vi "Pump Settings Dialog.vi"(8 "error in (no error)":errorcluster, 10 "Message Queues":T17, 11 "Pump Module State Cluster In":T1={"Pump Module Config"={"GUID"="", "Drop Coords"={"Horizontal"=0, "Vertical"=0}, "Process Name"="", "Queue Name"="", "Settings"={"Cycle Period"=500.0, "Manual Entry"=0.0, "Output Device"=enum."Default", "Ismatech"={"VISA resource name"="", "Simulated?"=TRUE, "Pump Number"=1.0, "Reverse?"=FALSE}, "Ismatech 3 Channel Settings"={"VISA resource name"="", "Pump Number"=1, "Channel Number"=0, "Simulated?"=TRUE, "Reverse?"=FALSE}, "Masterflex"={"VISA resource name"="", "Simulated?"=TRUE, "Pump Number"=1.0, "Reverse?"=FALSE}, "VICI Settings"={"VISA resource name"="", "Simulated?"=TRUE, "Pump Letter"="", "Reverse?"=FALSE}, "Tacmina Settings"={"Analog DAQ Task"="", "Digital DAQ Task"=""}, "KNF SIMDOS Settings"={"VISA resource name"="", "Simulated?"=TRUE}, "ASIA Pump C"={"ASIA Pump #"=0, "channel"=0, "Simulated"=FALSE}, "FLOM Settings"={"VISA resource name"="", "Simulated?"=TRUE, "Pump Number"=0.0}, "SSI PR/LD Settings"={"VISA resource name"="", "Simulated?"=FALSE}, "SSI P40 Settings"={"VISA resource name"="", "Simulated?"=FALSE}, "Masterflex 75211 Settings"={"Analog DAQ Task"="", "Digital DAQ Task"=""}, "Pump Calibration File"=path "", "Calibration Slope"=0.0, "Calibration Y Intercept"=0.0, "Pump Cal Enum"=0}, "Load Count"=0}, "State"=enum."Idle", "Start Time"=timestamp(0 s since 1904-01-01), "Current Time"=timestamp(0 s since 1904-01-01), "First Iteration"=FALSE, "Data"={"Pump Speed"=0.0}, "Process Name"="", "Pump On?"=FALSE} {"Pump Module Config"."Settings"."Ismatech 3 Channel Settings"."Channel Number" min=0 max=3; "Pump Module Config"."Settings"."Ismatech 3 Channel Settings"."Pump Number" min=1; "Pump Module Config"."Settings"."ASIA Pump C"."channel" min=0 max=1 step=1; "Pump Module Config"."Settings"."Masterflex"."Pump Number" min=1.0 max=20.0 step=1.0; "Pump Module Config"."Settings"."Ismatech"."Pump Number" min=1.0 max=20.0 step=1.0}) -> (0 "error out":errorcluster, 1 "Cancelled?":bool=TRUE, 2 "UI Refresh Needed?":bool, 3 "Pump Module Config Out":T2={"GUID"="", "Drop Coords"={"Horizontal"=0, "Vertical"=0}, "Process Name"="", "Queue Name"="", "Settings"={"Cycle Period"=0.0, "Manual Entry"=0.0, "Output Device"=enum."Default", "Ismatech"={"VISA resource name"="", "Simulated?"=FALSE, "Pump Number"=0.0, "Reverse?"=FALSE}, "Ismatech 3 Channel Settings"={"VISA resource name"="", "Pump Number"=1, "Channel Number"=0, "Simulated?"=TRUE, "Reverse?"=FALSE}, "Masterflex"={"VISA resource name"="", "Simulated?"=FALSE, "Pump Number"=0.0, "Reverse?"=FALSE}, "VICI Settings"={"VISA resource name"="", "Simulated?"=FALSE, "Pump Letter"="", "Reverse?"=FALSE}, "Tacmina Settings"={"Analog DAQ Task"="", "Digital DAQ Task"=""}, "KNF SIMDOS Settings"={"VISA resource name"="", "Simulated?"=TRUE}, "ASIA Pump C"={"ASIA Pump #"=0, "channel"=0, "Simulated"=FALSE}, "FLOM Settings"={"VISA resource name"="", "Simulated?"=TRUE, "Pump Number"=0.0}, "SSI PR/LD Settings"={"VISA resource name"="", "Simulated?"=FALSE}, "SSI P40 Settings"={"VISA resource name"="", "Simulated?"=FALSE}, "Masterflex 75211 Settings"={"Analog DAQ Task"="", "Digital DAQ Task"=""}, "Pump Calibration File"=path "", "Calibration Slope"=0.0, "Calibration Y Intercept"=0.0, "Pump Cal Enum"=0}, "Load Count"=0} {"Settings"."Ismatech 3 Channel Settings"."Channel Number" min=0 max=3; "Settings"."Ismatech 3 Channel Settings"."Pump Number" min=1; "Settings"."ASIA Pump C"."channel" min=0 max=1 step=1; "Settings"."Masterflex"."Pump Number" min=1.0 max=20.0 step=1.0; "Settings"."Ismatech"."Pump Number" min=1.0 max=20.0 step=1.0})   [LabVIEW 2018, in "Pump Module.lvlib"]
doc: "Dialog for selecting user specified settings."
uses:
  Pump Module.lvlib
  Pump Dialog Config and Start Stop Buttons.ctl
  Ismatec ISM 831C/Controls/Ismatech ISM831C Settings Cluster.ctl
  Masterflex 7550-30/Controls/Settings Cluster.ctl
  VICI M50 Party Mode/Settings Cluster.ctl
  Measure Instrument/PID 2 Output Enum.ctl
  Tacmina QI/Tacmina QI DAQ Setting.ctl
  KNF Pump/Settings Cluster plus SIMDOS.ctl
  ASIA Pump/Pump Settings.ctl
  FLOM Pump/Settings Cluster.ctl
  SSI PR Class/SSI PR or LD Settings Cluster.ctl
  Masterflex 75211/Masterflex 75211 DAQ Setting.ctl
  SSI PR Class/SSI P40 Settings Cluster.ctl
  Ismatec 78001/Ismatec 4083.ctl
  All Message Queues.ctl
  support/Message Queue/Message Cluster.ctl
  Pump Module Config Cluster.ctl
  <vilib>/Utility/miscctls.llb/LVPoint32TypeDef.ctl
  Pump Module Settings Cluster.ctl
  Pump Module State Cluster.ctl
  Measure Instrument/State Enum.ctl
  support/Message Queue/Enqueue Message (Single).vi
  <vilib>/Utility/xml.llb/Write to XML File(string).vi
  <vilib>/Utility/file.llb/Read Delimited Spreadsheet (string).vi
  Settings/Settings.lvlib
  support/Support Library.lvlib
  Masterflex 7550-30/Masterflex 7550-30.lvlib
  Ismatec ISM 831C/Ismatec ISM 831C.lvlib
  Tacmina QI/Tacmina QI.lvlib
  KNF Pump/KNF SIMDOS.lvlib
  VICI M50 Party Mode/VICI M6 M50 Party Mode.lvlib
  support/Message Queue/Message Queue.lvlib
  FLOM Pump/FLOM Pump.lvlib
  SSI PR Class/SSI PR or LD Pump.lvlib
  Masterflex 75211/Masterflex 75211.lvlib
  SSI PR Class/SSI P40 Pump.lvlib
  Ismatec 78001/Ismatec 4308.lvlib
  ASIA Pump.lvlib
  Measure Instrument/Feed Module Engine.lvlib
panel:
  in  "OK Button 2":bool
  in  "Module Name":string
  out "FLOM VISA Chosen":bool
  out "FLOM Number Chosen":bool
  in  "Pump Settings":T18={"Pump Configuration"={"Cycle Period"=500.0, "Ismatech"={"VISA resource name"="", "Simulated?"=FALSE, "Pump Number"=1.0, "Reverse?"=FALSE}, "Masterflex"={"VISA resource name"="", "Simulated?"=FALSE, "Pump Number"=1.0, "Reverse?"=FALSE}, "Pump %"=0.0, "VICI Settings"={"VISA resource name"="", "Simulated?"=FALSE, "Pump Letter"="", "Reverse?"=FALSE}, "Output Device"=enum."Default", "Tacmina Settings"={"Analog DAQ Task"="", "Digital DAQ Task"=""}, "KNF SIMDOS Settings"={"VISA resource name"="", "Simulated?"=FALSE}, "ASIA Pump C"={"ASIA Pump #"=-1, "channel"=-1, "Simulated"=FALSE}, "FLOM Settings"={"VISA resource name"="", "Simulated?"=FALSE, "Pump Number"=1.0}, "Pump Calibration"=0, "SSI PR/LD Settings"={"VISA resource name"="", "Simulated?"=FALSE}, "Masterflex 75211 Settings"={"Analog DAQ Task"="", "Digital DAQ Task"=""}, "SSI P40 Settings"={"VISA resource name"="", "Simulated?"=FALSE}, "Ismatech 3 Channel Settings"={"VISA resource name"="", "Pump Number"=0, "Channel Number"=0, "Simulated?"=FALSE, "Reverse?"=FALSE}}, "Stop"=FALSE, "Start"=FALSE} {"Pump Configuration"."Ismatech 3 Channel Settings"."Channel Number" min=0 max=3; "Pump Configuration"."Ismatech 3 Channel Settings"."Pump Number" min=1; "Pump Configuration"."ASIA Pump C"."channel" min=-1 max=1 step=1; "Pump Configuration"."Ismatech"."Pump Number" min=1.0 max=20.0 step=1.0; "Pump Configuration"."Masterflex"."Pump Number" min=1.0 max=20.0 step=1.0}
  in  "Cancel Button":bool
  in  "OK Button":bool
  # "Non visible portion of dialog (needed for connector pane)."
  # "Output Instruments"
  # "Output Instruments"
  # "Output Instruments"
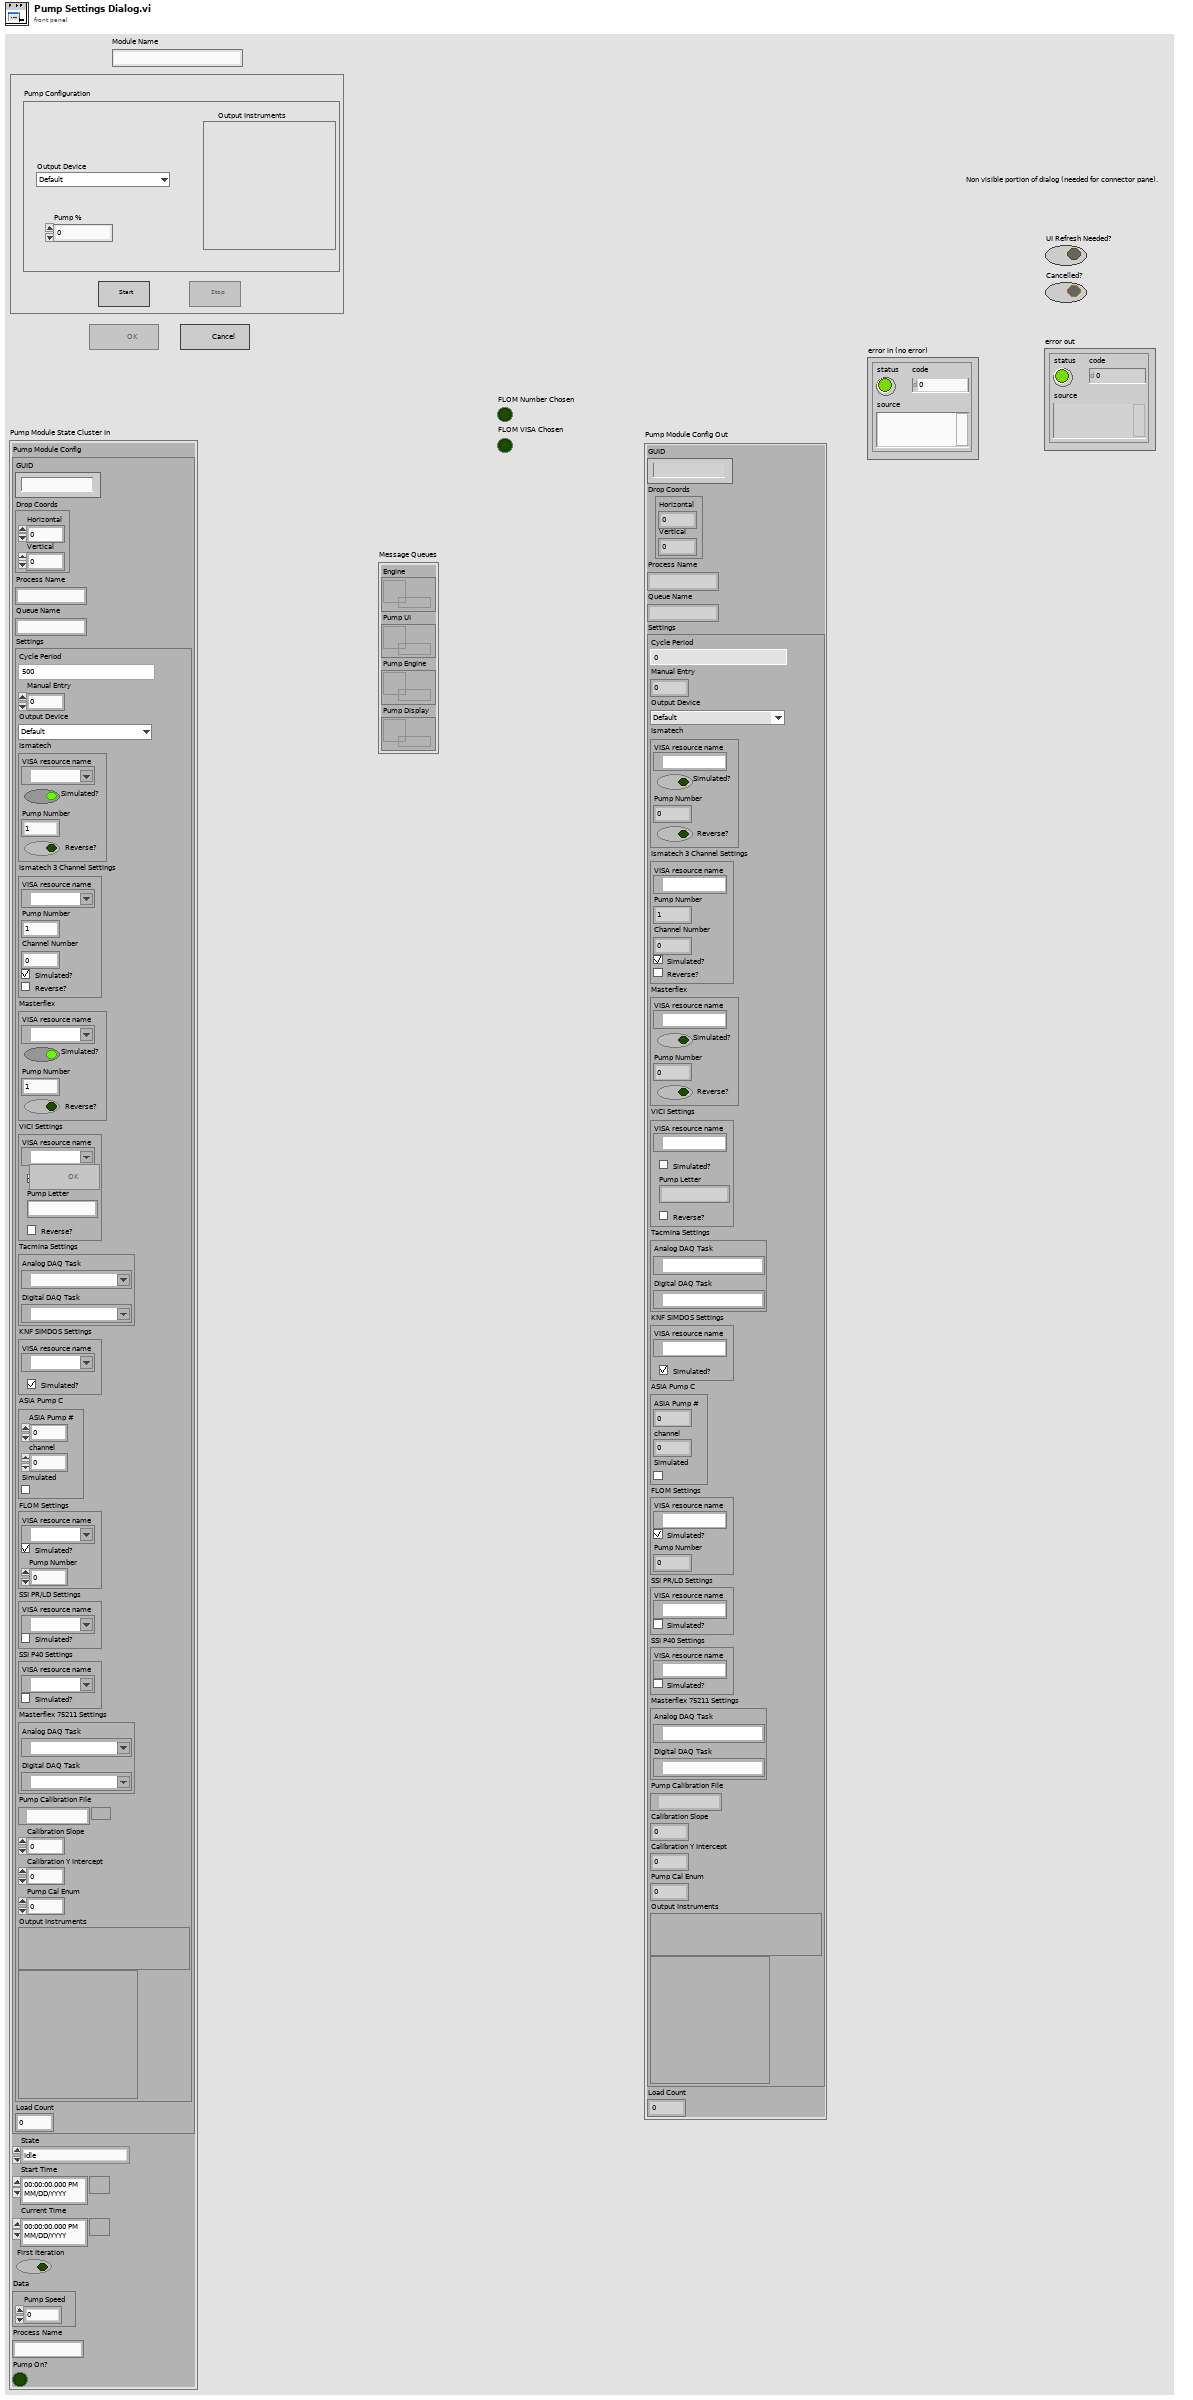
[diagram p1: front panel]
types:
  T1 = typedef "Pump Module.lvlib/Pump Module State Cluster.ctl" = cluster{"Pump Module Config":T2, "State":T16, "Start Time":timestamp, "Current Time":timestamp, "First Iteration":bool, "Data":cluster{"Pump Speed":dbl}, "Process Name":string, "Pump On?":bool}
  T2 = typedef "Pump Module.lvlib/Pump Module Config Cluster.ctl" = cluster{"GUID":string, "Drop Coords":T3, "Process Name":string, "Queue Name":string, "Settings":T4, "Load Count":i32}
  T3 = typedef "LVPoint32TypeDef.ctl" = cluster{"Horizontal":i32, "Vertical":i32}
  T4 = typedef "Pump Module.lvlib/Pump Module Settings Cluster.ctl" = cluster{"Cycle Period":dbl, "Manual Entry":dbl, "Output Device":T5, "Ismatech":T6, "Ismatech 3 Channel Settings":T7, "Masterflex":T8, "VICI Settings":T9, "Tacmina Settings":T10, "KNF SIMDOS Settings":T11, "ASIA Pump C":T12, "FLOM Settings":T13, "SSI PR/LD Settings":T14, "SSI P40 Settings":T14, "Masterflex 75211 Settings":T15, "Pump Calibration File":path, "Calibration Slope":dbl, "Calibration Y Intercept":dbl, "Pump Cal Enum":u16}
  T5 = typedef "PID 2 Output Enum.ctl" = enum16{"Default", "Ismatec ISM 4308", "Ismatec ISM 831C", "Masterflex 7550-30", "VICI", "Tacmina QI", "KNF SIMDOS", "ASIA Type C", "FLOM UI-22-11", "SSI PR/LD", "SSI P40", "Masterflex 75211-70"}
  T6 = typedef "Ismatec ISM 831C.lvlib/Ismatech ISM831C Settings Cluster.ctl" = cluster{"VISA resource name":refnum<visa-resource-name>, "Simulated?":bool, "Pump Number":dbl, "Reverse?":bool}
  T7 = typedef "Ismatec 4308.lvlib/Ismatec 4083.ctl" = cluster{"VISA resource name":refnum<visa-resource-name>, "Pump Number":i16, "Channel Number":i16, "Simulated?":bool, "Reverse?":bool}
  T8 = typedef "Masterflex 7550-30.lvlib/Settings Cluster.ctl" = cluster{"VISA resource name":refnum<visa-resource-name>, "Simulated?":bool, "Pump Number":dbl, "Reverse?":bool}
  T9 = typedef "VICI M6 M50 Party Mode.lvlib/Settings Cluster.ctl" = cluster{"VISA resource name":refnum<visa-resource-name>, "Simulated?":bool, "Pump Letter":string, "Reverse?":bool}
  T10 = typedef "Tacmina QI.lvlib/Tacmina QI DAQ Setting.ctl" = cluster{"Analog DAQ Task":refnum<k21>, "Digital DAQ Task":refnum<k21>}
  T11 = typedef "KNF SIMDOS.lvlib/Settings Cluster plus SIMDOS.ctl" = cluster{"VISA resource name":refnum<visa-resource-name>, "Simulated?":bool}
  T12 = typedef "ASIA Pump.lvlib/Pump Settings.ctl" = cluster{"ASIA Pump #":i32, "channel":i32, "Simulated":bool}
  T13 = typedef "FLOM Pump.lvlib/Settings Cluster.ctl" = cluster{"VISA resource name":refnum<visa-resource-name>, "Simulated?":bool, "Pump Number":dbl}
  T14 = typedef "SSI PR or LD Pump.lvlib/SSI PR or LD Settings Cluster.ctl" = cluster{"VISA resource name":refnum<visa-resource-name>, "Simulated?":bool}
  T15 = typedef "Masterflex 75211.lvlib/Masterflex 75211 DAQ Setting.ctl" = cluster{"Analog DAQ Task":refnum<k21>, "Digital DAQ Task":refnum<k21>}
  T16 = typedef "Feed Module.lvlib/Feed Module Engine.lvlib/State Enum.ctl" = enum16{"Measuring", "Idle", "Paused"}
  T17 = typedef "Pump Module.lvlib/All Message Queues.ctl" = cluster{"Engine":refnum<queue>, "Pump UI":refnum<queue>, "Pump Engine":refnum<queue>, "Pump Display":refnum<queue>}
  T18 = typedef "Pump Module.lvlib/Pump Dialog Config and Start Stop Buttons.ctl" = cluster{"Pump Configuration":cluster{"Cycle Period":dbl, "Ismatech":T6, "Masterflex":T8, "Pump %":dbl, "VICI Settings":T9, "Output Device":T5, "Tacmina Settings":T10, "KNF SIMDOS Settings":T11, "ASIA Pump C":T12, "FLOM Settings":T13, "Pump Calibration":u16, "SSI PR/LD Settings":T14, "Masterflex 75211 Settings":T15, "SSI P40 Settings":T19, "Ismatech 3 Channel Settings":T7}, "Stop":bool, "Start":bool}
  T19 = typedef "SSI P40 Pump.lvlib/SSI P40 Settings Cluster.ctl" = cluster{"VISA resource name":refnum<visa-resource-name>, "Simulated?":bool}
  T20 = cluster{"Cycle Period":dbl, "Ismatech":T6, "Masterflex":T8, "Pump %":dbl, "VICI Settings":T9, "Output Device":T5, "Tacmina Settings":T10, "KNF SIMDOS Settings":T11, "ASIA Pump C":T12, "FLOM Settings":T13, "Pump Calibration":u16, "SSI PR/LD Settings":T14, "Masterflex 75211 Settings":T15, "SSI P40 Settings":T19, "Ismatech 3 Channel Settings":T7}
  T21 = cluster{"Pump Configuration":cluster{"Cycle Period":dbl, "Ismatech":T6, "Masterflex":T8, "Pump %":dbl, "VICI Settings":T9, "Output Device":T5, "Tacmina Settings":T10, "KNF SIMDOS Settings":T11, "ASIA Pump C":T12, "FLOM Settings":T13, "Pump Calibration":u16, "SSI PR/LD Settings":T14, "Masterflex 75211 Settings":T15, "SSI P40 Settings":T19, "Ismatech 3 Channel Settings":T7}, "Stop":bool, "Start":bool}
  T22 = enum8{"Enabled", "Disabled", "Disabled and Grayed Out"}
  T23 = typedef "Ismatec 78001.lvlib/Ismatec 78001.ctl" = cluster{"VISA resource name":refnum<visa-resource-name>, "Pump Number":i16, "Channel Number":i16, "Simulated?":bool, "Reverse?":bool}
  T24 = cluster{"Cycle Period":dbl, "Ismatech":T6, "Masterflex":T8, "Pump %":dbl, "VICI Settings":T9, "Output Device":T5, "Tacmina Settings":T10, "KNF SIMDOS Settings":T11, "ASIA Pump C":T12, "FLOM Settings":T13, "Pump Calibration":u16, "SSI PR/LD Settings":T14, "Masterflex 75211 Settings":T15, "SSI P40 Settings":T19, "Ismatech 3 Channel Settings":T23}
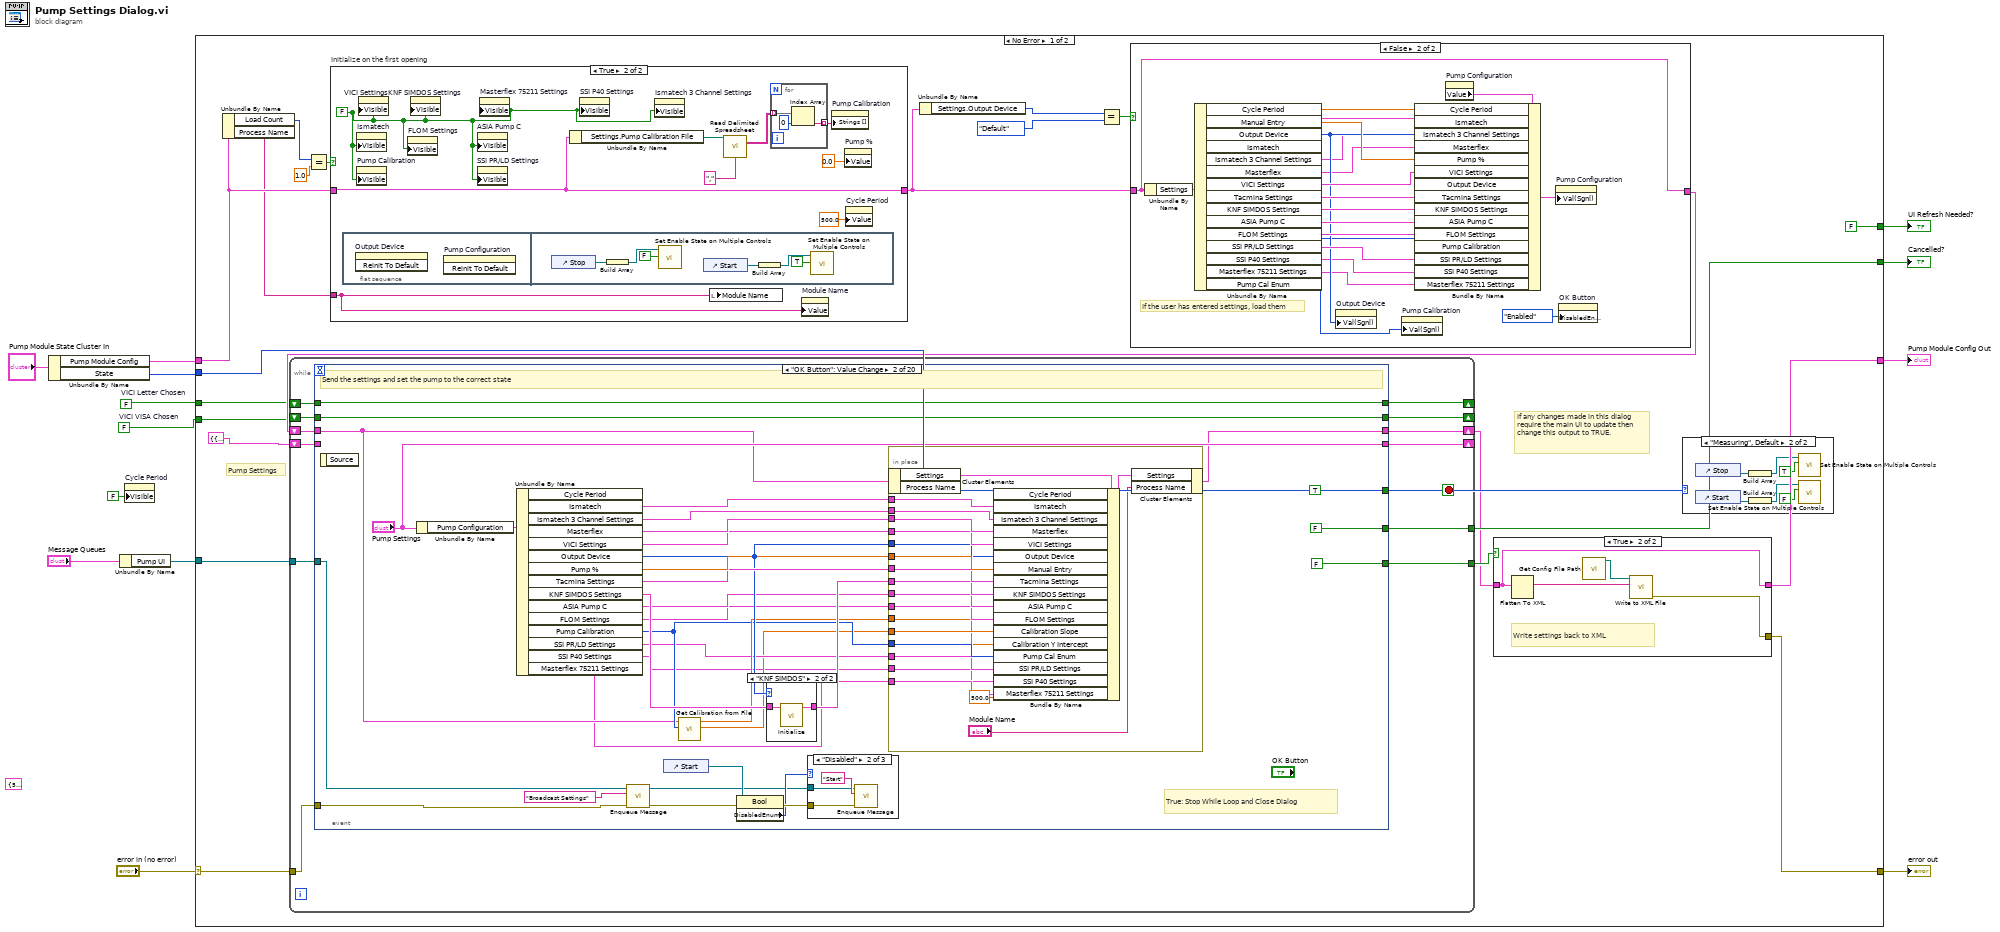
[diagram p0: block diagram]
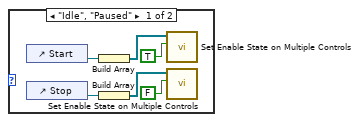
[diagram p2: hidden frame]
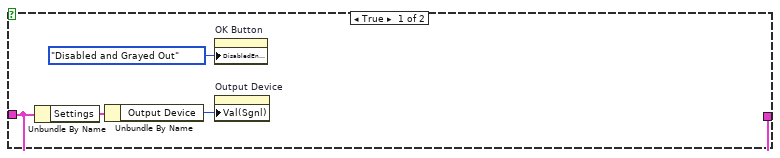
[diagram p3: hidden frame]
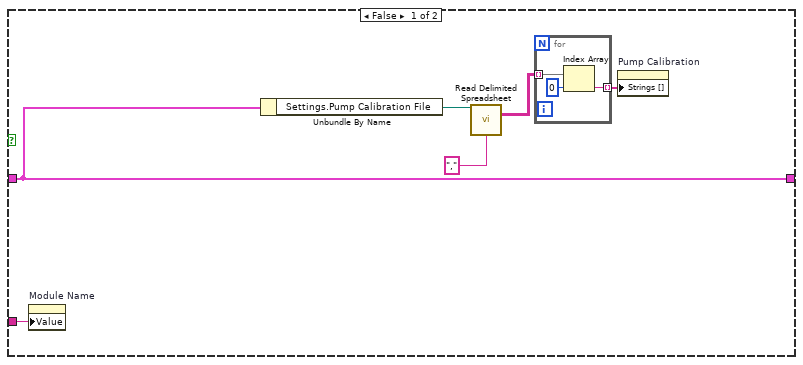
[diagram p4: hidden frame]
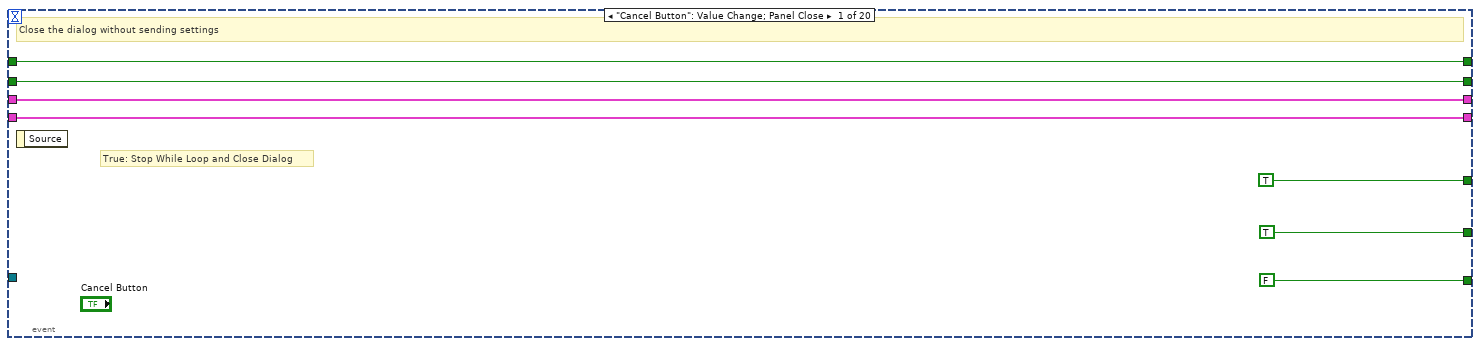
[diagram p5: hidden frame]
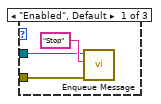
[diagram p6: hidden frame]
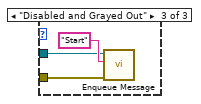
[diagram p7: hidden frame]
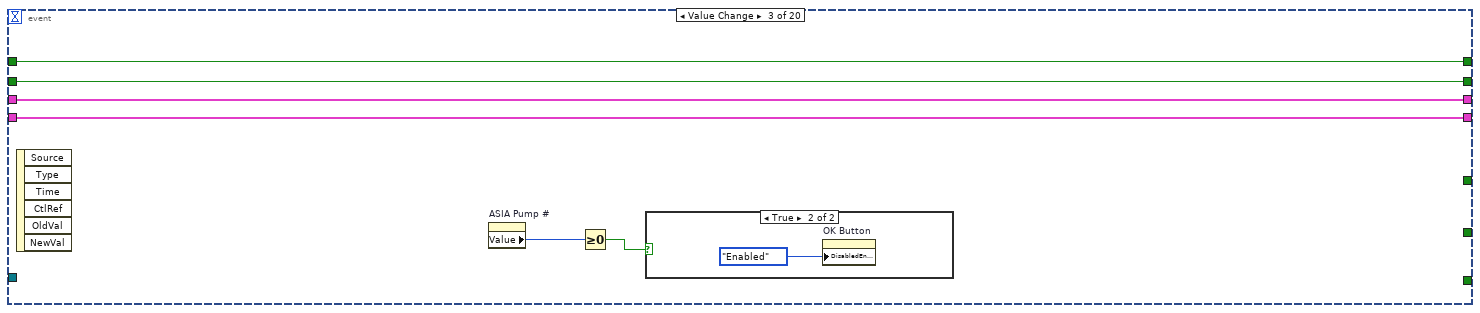
[diagram p9: hidden frame]
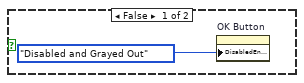
[diagram p10: hidden frame]
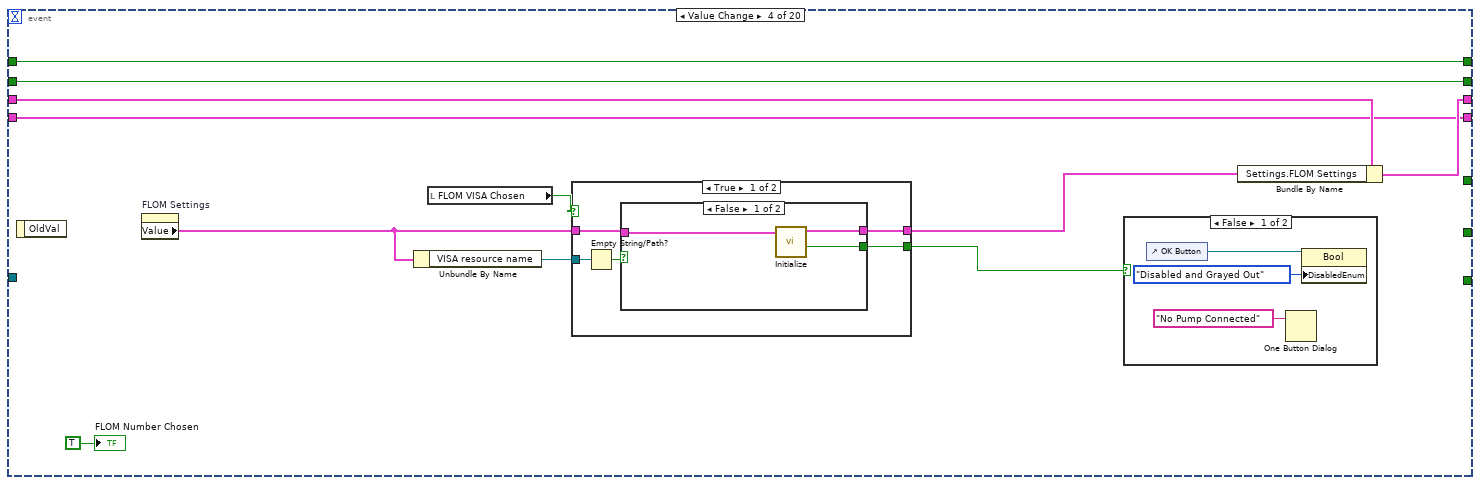
[diagram p11: hidden frame]
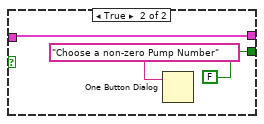
[diagram p12: hidden frame]
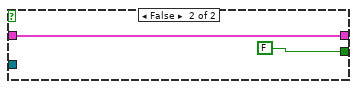
[diagram p13: hidden frame]
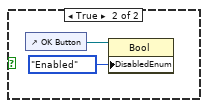
[diagram p14: hidden frame]
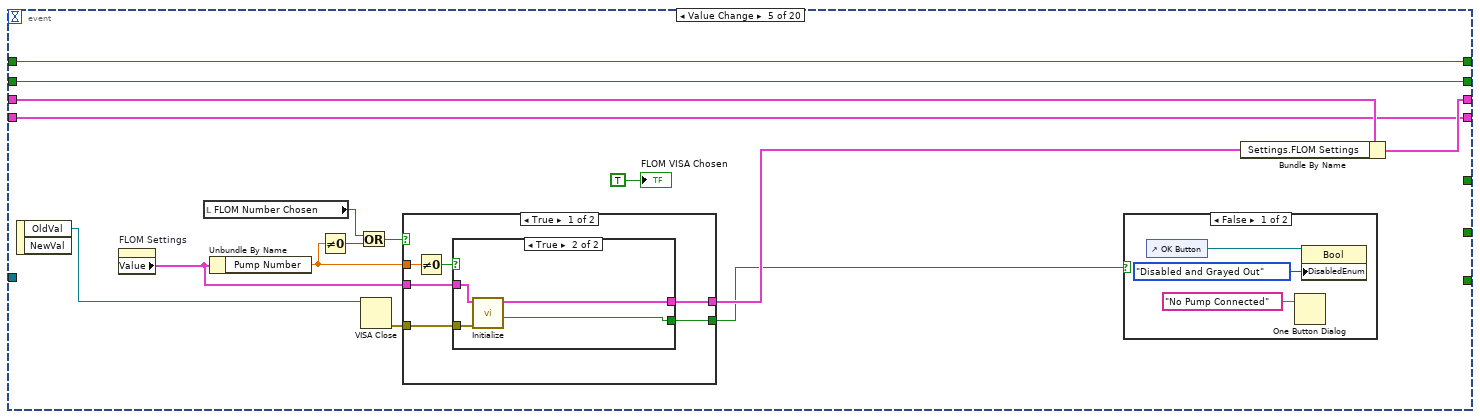
[diagram p15: hidden frame]
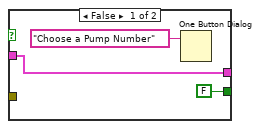
[diagram p16: hidden frame]
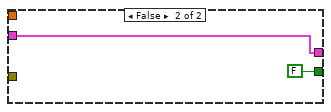
[diagram p17: hidden frame]
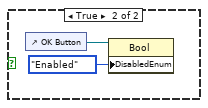
[diagram p18: hidden frame]
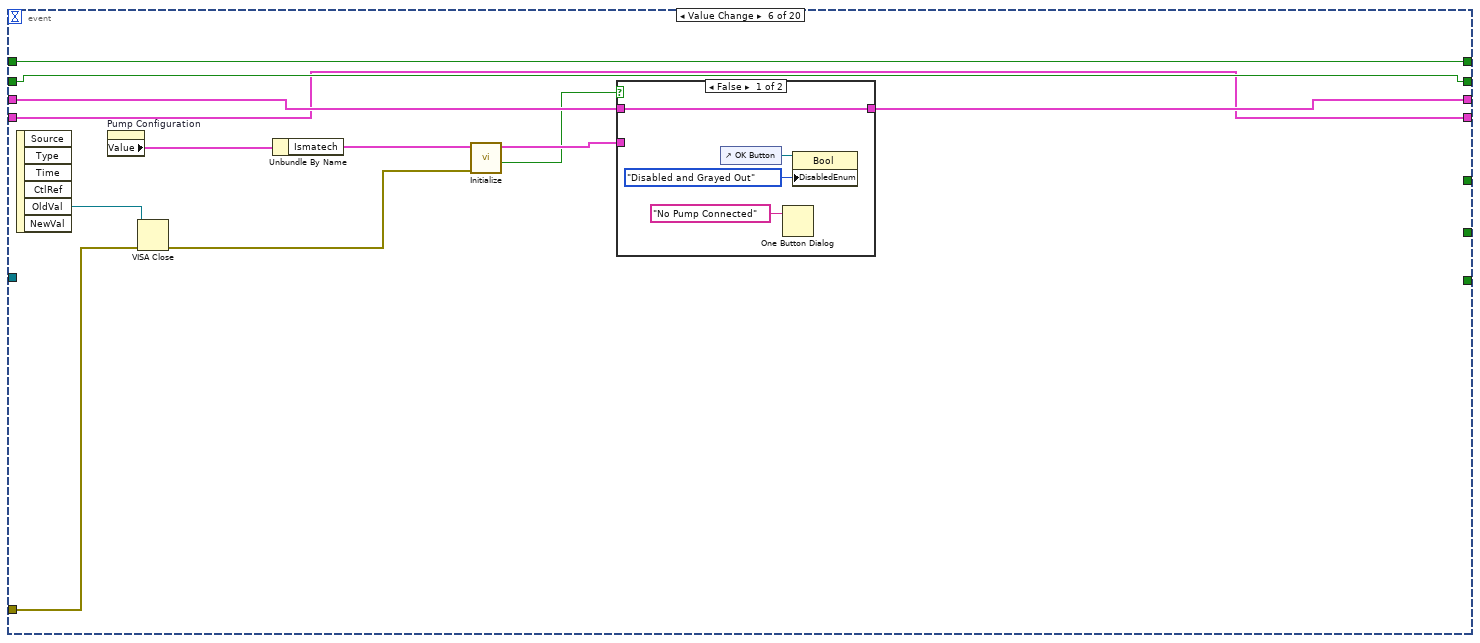
[diagram p19: hidden frame]
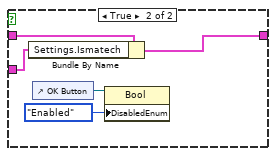
[diagram p20: hidden frame]
diagram:
  (unwired) T20 {"Cycle Period"=500.0, "Ismatech"={"VISA resource name"="", "Simulated?"=FALSE, "Pump Number"=1.0, "Reverse?"=FALSE}, "Masterflex"={"VISA resource name"="", "Simulated?"=FALSE, "Pump Number"=1.0, "Reverse?"=FALSE}, "Pump %"=0.0, "VICI Settings"={"VISA resource name"="", "Simulated?"=FALSE, "Pump Letter"="", "Reverse?"=FALSE}, "Output Device"=enum."Default", "Tacmina Settings"={"Analog DAQ Task"="", "Digital DAQ Task"=""}, "KNF SIMDOS Settings"={"VISA resource name"="", "Simulated?"=FALSE}, "ASIA Pump C"={"ASIA Pump #"=-1, "channel"=-1, "Simulated"=FALSE}, "FLOM Settings"={"VISA resource name"="", "Simulated?"=FALSE, "Pump Number"=1.0}, "Pump Calibration"=0, "SSI PR/LD Settings"={"VISA resource name"="", "Simulated?"=FALSE}, "Masterflex 75211 Settings"={"Analog DAQ Task"="", "Digital DAQ Task"=""}, "SSI P40 Settings"={"VISA resource name"="", "Simulated?"=FALSE}, "Ismatech 3 Channel Settings"={"VISA resource name"="", "Pump Number"=0, "Channel Number"=0, "Simulated?"=FALSE, "Reverse?"=FALSE}} ("Pump Configuration")
  w2 = FALSE  # VICI VISA Chosen
  w3 = FALSE  # VICI Letter Chosen
  n1 = Unbundle By Name("Pump Module State Cluster In") -> ("Pump Module Config"=w5:T2, "State"=w4:T16)
  n2 = Unbundle By Name("Message Queues") -> ("Pump UI"=w10:refnum<queue>)
  n3 = property on="Cycle Period" class="DigNum (strict)"("Visible"=FALSE) -> ()  [unwired: 2 in, 2 out]
  n4 = case shown="No Error" "error in (no error)" {
    selector: "error in (no error)" -> [w30 w704]
    tunnel: [w32 w704] -> w13
    tunnel: w5 -> [w29 w702]
    tunnel: [w33 w702] -> w7
    tunnel: [FALSE ("UI Refresh Needed?") _] -> w12
    tunnel: [w34 TRUE ("UI Refresh Needed?")] -> w11
    tunnel: w10 -> [w31 _]
    tunnel: w4 -> [w28 _]
    tunnel: w3 -> [w21 _]
    tunnel: w2 -> [w20 _]
    frame No Error {
      # "Pump Settings"
      # "If any changes made in this dialog require the main UI to update then change this output to TRUE."
      n5 = Unbundle By Name(w29) -> ("Load Count"=w27:i32, "Process Name"=w15:string)
      n6 = Equal?(x=w27, y=1.0) -> (x = y?=w25:bool)
      n7 = case "Initialize on the first opening" shown="True" w25 {
        tunnel: w29 -> [w73 w89]
        tunnel: [w73 w89] -> w19
        tunnel: w15 -> [w72 w82]
        frame False {
          n8 = property on="Module Name" class="Str"("Value"=w72) -> ()  [unwired: 2 in, 2 out]
          n9 = Unbundle By Name(w73) -> ("Settings.Pump Calibration File"=w77:path)
          n10 = call-poly <vilib>:"Read Delimited Spreadsheet.vi"("file path (dialog if empty)"=w77, "delimiter (\\t)"="," ("delimiter (\\t)")) -> ("all rows"=w76:string[][])  [unwired: 8 in, 5 out]
          n11 = for {
            tunnel: w76 -> [w79] mode=indexing
            tunnel: [w78] -> w75 mode=indexing
            n12 = Index Array(array=w79, index=0) -> (element=w78:string)
          }
          n13 = property on="Pump Calibration" class="Ring (strict)"("Strings []"=w75) -> ()  [unwired: 2 in, 2 out]
        }
        frame True {
          w81 = FALSE ("Visible")
          n14 = flat-sequence {
            frame #0 {
              n15 = invoke on="Output Device" class="Enum (strict)" method="Reinit To Default"() -> ()  [unwired: 3 in, 3 out]
              n16 = invoke on="Pump Configuration" class="Clust (strict)" method="Reinit To Default"() -> ()  [unwired: 3 in, 3 out]
            }
            frame #1 {
              n17 = control-ref of="Stop"() -> (w95:refnum<vi>)
              n18 = Build Array(w95) -> (w94:refnum<vi>[])
              n19 = call "Set Enable State on Multiple Controls.vi"("Enable?"=FALSE, "Controls"=w94) -> ()  [unwired: 10 in]
              n20 = control-ref of="Start"() -> (w92:refnum<vi>)
              n21 = Build Array(w92) -> (w91:refnum<vi>[])
              n22 = call "Set Enable State on Multiple Controls.vi"("Enable?"=TRUE, "Controls"=w91) -> ()  [unwired: 10 in]
            }
          }
          n23 = property on="Ismatech" class="Clust (strict)"("Visible"=w81) -> ()  [unwired: 2 in, 2 out]
          n24 = property on="Pump Calibration" class="Ring (strict)"("Visible"=w81) -> ()  [unwired: 2 in, 2 out]
          n25 = property on="VICI Settings" class="Clust (strict)"("Visible"=w81) -> ()  [unwired: 2 in, 2 out]
          n26 = property on="FLOM Settings" class="Clust (strict)"("Visible"=w81) -> ()  [unwired: 2 in, 2 out]
          n27 = property on="KNF SIMDOS Settings" class="Clust (strict)"("Visible"=w81) -> ()  [unwired: 2 in, 2 out]
          n28 = property on="ASIA Pump C" class="Clust (strict)"("Visible"=w81) -> ()  [unwired: 2 in, 2 out]
          n29 = property on="SSI PR/LD Settings" class="Clust (strict)"("Visible"=w81) -> ()  [unwired: 2 in, 2 out]
          n30 = property on="Masterflex 75211 Settings" class="Clust (strict)"("Visible"=w81) -> ()  [unwired: 2 in, 2 out]
          n31 = Unbundle By Name(w89) -> ("Settings.Pump Calibration File"=w86:path)
          n32 = property on="SSI P40 Settings" class="Clust (strict)"("Visible"=w81) -> ()  [unwired: 2 in, 2 out]
          n33 = property on="Ismatech 3 Channel Settings" class="Clust (strict)"("Visible"=w81) -> ()  [unwired: 2 in, 2 out]
          n34 = local write "Module Name"(w82) -> ()
          n35 = call-poly <vilib>:"Read Delimited Spreadsheet.vi"("file path (dialog if empty)"=w86, "delimiter (\\t)"="," ("delimiter (\\t)")) -> ("all rows"=w84:string[][])  [unwired: 8 in, 5 out]
          n36 = for {
            tunnel: w84 -> [w97] mode=indexing
            tunnel: [w96] -> w83 mode=indexing
            n37 = Index Array(array=w97, index=0) -> (element=w96:string)
          }
          n38 = property on="Module Name" class="Str"("Value"=w82) -> ()  [unwired: 2 in, 2 out]
          n39 = property on="Pump Calibration" class="Ring (strict)"("Strings []"=w83) -> ()  [unwired: 2 in, 2 out]
          n40 = property on="Pump %" class="DigNum (strict)"("Value"=0.0) -> ()  [unwired: 2 in, 2 out]
          n41 = property on="Cycle Period" class="DigNum (strict)"("Value"=500.0) -> ()  [unwired: 2 in, 2 out]
        }
      }
      n42 = Unbundle By Name(w19) -> ("Settings.Output Device"=w17:T5)
      n43 = Equal?(x=w17, y=PID_2_Output_Enum."Default" ("Settings.Output Device")) -> (x = y?=w16:bool)
      n44 = case shown="False" w16 {
        tunnel: w19 -> [w49 w62]
        tunnel: [w49 w62] -> w22
        frame True {
          n45 = Unbundle By Name(w49) -> ("Settings"=w51:T4)
          n46 = Unbundle By Name(w51) -> ("Output Device"=w50:T5)
          n47 = property on="OK Button" class="Bool"("DisabledEnum"=T22."Disabled and Grayed Out" ("Disabled")) -> ()  [unwired: 2 in, 2 out]
          n48 = property on="Output Device" class="Enum (strict)"("Val(Sgnl)"=w50) -> ()  [unwired: 2 in, 2 out]
        }
        frame False {
          # "If the user has entered settings, load them"
          n49 = Unbundle By Name(w62) -> ("Settings"=w69:T4)
          n50 = Unbundle By Name(w69) -> ("Cycle Period"=w71:dbl, "Manual Entry"=w61:dbl, "Output Device"=w57:T5, "Ismatech"=w60:T6, "Ismatech 3 Channel Settings"=w52:T7, "Masterflex"=w54:T8, "VICI Settings"=w59:T9, "Tacmina Settings"=w68:T10, "KNF SIMDOS Settings"=w67:T11, "ASIA Pump C"=w66:T12, "FLOM Settings"=w65:T13, "SSI PR/LD Settings"=w58:T14, "SSI P40 Settings"=w56:T14, "Masterflex 75211 Settings"=w55:T15, "Pump Cal Enum"=w53:u16)
          n51 = property on="Output Device" class="Enum (strict)"("Val(Sgnl)"=w57) -> ()  [unwired: 2 in, 2 out]
          n52 = property on="Pump Calibration" class="Ring (strict)"("Val(Sgnl)"=w53) -> ()  [unwired: 2 in, 2 out]
          n53 = property on="Pump Configuration" class="Clust (strict)"() -> ("Value"=w63:T24)  [unwired: 2 in, 2 out]
          n54 = Bundle By Name(cluster=w63, "Cycle Period"=w71, "Ismatech"=w60, "Ismatech 3 Channel Settings"=w52, "Masterflex"=w54, "Pump %"=w61, "VICI Settings"=w59, "Output Device"=w57, "Tacmina Settings"=w68, "KNF SIMDOS Settings"=w67, "ASIA Pump C"=w66, "FLOM Settings"=w65, "Pump Calibration"=w53, "SSI PR/LD Settings"=w58, "SSI P40 Settings"=w56, "Masterflex 75211 Settings"=w55) -> (w70:T24)
          n55 = property on="Pump Configuration" class="Clust (strict)"("Val(Sgnl)"=w70) -> ()  [unwired: 2 in, 2 out]
          n56 = property on="OK Button" class="Bool"("DisabledEnum"=T22."Enabled" ("Disabled")) -> ()  [unwired: 2 in, 2 out]
        }
      }
      n57 = while {
        tunnel: [w111] -> w24
        tunnel: [w109] -> w34
        tunnel: w31 -> [w107]
        tunnel: w30 -> [w106]
        shift-right: [w108] -> w23
        shift-left: w22 -> [w105]
        shift-right: [w104] -> _
        shift-left: w21 -> [w103]
        shift-right: [w102] -> _
        shift-left: w20 -> [w101]
        shift-right: [w100] -> _
        shift-left: T21 {"Pump Configuration"={"Cycle Period"=500.0, "Ismatech"={"VISA resource name"="", "Simulated?"=FALSE, "Pump Number"=1.0, "Reverse?"=FALSE}, "Masterflex"={"VISA resource name"="", "Simulated?"=FALSE, "Pump Number"=1.0, "Reverse?"=FALSE}, "Pump %"=0.0, "VICI Settings"={"VISA resource name"="", "Simulated?"=FALSE, "Pump Letter"="", "Reverse?"=FALSE}, "Output Device"=enum."Default", "Tacmina Settings"={"Analog DAQ Task"="", "Digital DAQ Task"=""}, "KNF SIMDOS Settings"={"VISA resource name"="", "Simulated?"=FALSE}, "ASIA Pump C"={"ASIA Pump #"=-1, "channel"=-1, "Simulated"=FALSE}, "FLOM Settings"={"VISA resource name"="", "Simulated?"=FALSE, "Pump Number"=1.0}, "Pump Calibration"=0, "SSI PR/LD Settings"={"VISA resource name"="", "Simulated?"=FALSE}, "Masterflex 75211 Settings"={"Analog DAQ Task"="", "Digital DAQ Task"=""}, "SSI P40 Settings"={"VISA resource name"="", "Simulated?"=FALSE}, "Ismatech 3 Channel Settings"={"VISA resource name"="", "Pump Number"=0, "Channel Number"=0, "Simulated?"=FALSE, "Reverse?"=FALSE}}, "Stop"=FALSE, "Start"=FALSE} ("Pump Settings") -> [w99]
        stop <- w110 stop-if-true
        n58 = event shown="[1] \"OK Button\": Value Change" {
          selector: _ -> [_ _ _ _ _ _ _ _ _ _ _ _ _ _ _ _ _ _ _ _]
          dyn-events: _ -> [_ _ _ _ _ _ _ _ _ _ _ _ _ _ _ _ _ _ _ _]
          timeout: _ -> [_ _ _ _ _ _ _ _ _ _ _ _ _ _ _ _ _ _ _ _]
          tunnel: [FALSE ("UI Refresh Needed?") FALSE ("UI Refresh Needed?") _ _ _ _ _ _ _ _ _ _ _ _ _ _ _ _ _ _] -> w111
          tunnel: [TRUE TRUE _ _ _ _ _ _ _ _ _ _ _ _ _ _ _ _ _ _] -> w110
          tunnel: [TRUE ("UI Refresh Needed?") FALSE ("UI Refresh Needed?") _ _ _ _ _ _ _ _ _ _ _ _ _ _ _ _ _ _] -> w109
          tunnel: w105 -> [w115 w123 w186 w203 w236 w263 w290 w335 w353 w372 w553 w573 w590 w605 w617 w637 w648 w670 w682 w695]
          tunnel: [w115 w122 w186 w202 w235 w262 w290 w334 w352 w371 w552 w572 w589 w604 w616 w637 w647 w670 w682 w695] -> w108
          tunnel: w107 -> [_ w149 _ _ _ _ _ _ _ _ _ _ _ _ _ _ _ _ _ _]
          tunnel: w106 -> [_ w148 _ _ _ w261 _ w333 w351 _ w551 w567 _ _ w615 _ w646 _ _ _]
          tunnel: [w113 w136 w190 w201 w234 w259 w288 w328 w349 w369 TRUE ("VICI VISA Chosen") TRUE ("VICI VISA Chosen") w587 w603 TRUE ("VICI VISA Chosen") TRUE ("VICI VISA Chosen") w645 w671 w680 w693] -> w104
          tunnel: w103 -> [w113 w136 w190 w201 w234 w259 w288 w328 w349 w369 _ _ w587 w603 _ _ w645 w671 w680 w693]
          tunnel: [w114 w137 w189 w200 w233 w260 w289 w329 w350 w370 w550 w571 w586 w602 w614 w640 TRUE ("VICI VISA Chosen") w672 w681 w694] -> w102
          tunnel: w101 -> [w114 w137 w189 w200 w233 w260 w289 w329 w350 w370 w550 w571 w586 w602 w614 w640 _ w672 w681 w694]
          tunnel: [w112 "Pump Settings" w188 w199 w232 w258 w287 w327 w348 w368 w548 w569 w585 w601 w612 w638 w643 w669 w679 w692] -> w100
          tunnel: w99 -> [w112 _ w188 w199 w232 w258 w287 w327 w348 w368 w548 w569 w585 w601 w612 w638 w643 w669 w679 w692]
          event "Cancel Button": Value Change; Panel Close {
            # "True: Stop While Loop and Close Dialog"
            # "Close the dialog without sending settings"
            n59 = event-data() -> ()  [unwired: 1 in, 1 out]
          }
          event "OK Button": Value Change {
            (unwired) cluster{"Stop":bool, "Start":bool} {"Stop"=FALSE, "Start"=FALSE} ("Pump Settings 2")
            (unwired) cluster{"Stop":bool, "Start":bool} {"Stop"=FALSE, "Start"=FALSE} ("Pump Settings")
            # "True: Stop While Loop and Close Dialog"
            # "Send the settings and set the pump to the correct state"
            n60 = event-data() -> ()  [unwired: 1 in, 1 out]
            n61 = Unbundle By Name("Pump Settings") -> ("Pump Configuration"=w147:T20)
            n62 = Unbundle By Name(w147) -> ("Ismatech"=w146:T6, "Ismatech 3 Channel Settings"=w119:T7, "Masterflex"=w145:T8, "VICI Settings"=w144:T9, "Output Device"=w141:T5, "Pump %"=w143:dbl, "Tacmina Settings"=w142:T10, "KNF SIMDOS Settings"=w140:T11, "ASIA Pump C"=w138:T12, "FLOM Settings"=w128:T13, "Pump Calibration"=w126:u16, "SSI PR/LD Settings"=w125:T14, "SSI P40 Settings"=w120:T19, "Masterflex 75211 Settings"=w121:T15)  [unwired: 1 out]
            n63 = call-poly "Enqueue Message.vi"("error in (no error)"=w148, "Message"="Broadcast Settings", "Message Queue"=w149) -> ("error out"=w130:errorcluster, "dup Message Queue"=w129:refnum<queue>)  [unwired: 7 in]
            n64 = control-ref of="Start"() -> (w133:refnum<vi>)
            n65 = call "Get Calibration from File.vi"("Pump Calibration"=w126, "Pump Module Config"=w123) -> ("Calibration Y Intercept"=w124:dbl, "Calibration Slope"=w127:dbl)  [unwired: 8 in]
            n66 = property class="Bool"(reference=w133, error in=w130) -> (error out=w134:errorcluster, "DisabledEnum"=w132:T22)  [unwired: 1 out]
            n67 = case shown="\"KNF SIMDOS\"" w141 {
              tunnel: w140 -> [w182 w184]
              tunnel: [w182 w183] -> w139
              frame "Default", Default {
              }
              frame "KNF SIMDOS" {
                n68 = call "Initialize.vi"("KNF Settings In"=w184) -> ("KNF Settings Out"=w183:T11)  [unwired: 7 in, 3 out]
              }
            }
            n69 = case shown="\"Disabled\"" w132 {
              tunnel: w134 -> [w174 w177 w180]
              tunnel: w129 -> [w173 w176 w179]
              frame "Enabled", Default {
                n70 = call-poly "Enqueue Message.vi"("error in (no error)"=w174, "Message"="Stop", "Message Queue"=w173) -> ()  [unwired: 7 in, 2 out]
              }
              frame "Disabled" {
                n71 = call-poly "Enqueue Message.vi"("error in (no error)"=w177, "Message"="Start", "Message Queue"=w176) -> ()  [unwired: 7 in, 2 out]
              }
              frame "Disabled and Grayed Out" {
                n72 = call-poly "Enqueue Message.vi"("error in (no error)"=w180, "Message"="Start", "Message Queue"=w179) -> ()  [unwired: 7 in, 2 out]
              }
            }
            n73 = in-place {
              in-place-border: w146 -> [w172]
              in-place-border: w145 -> [w171]
              in-place-border: w144 -> [w170]
              in-place-border: w143 -> [w169]
              in-place-border: w142 -> [w168]
              in-place-border: w141 -> [w167]
              in-place-border: w139 -> [w166]
              in-place-border: w138 -> [w165]
              in-place-border: w128 -> [w163]
              in-place-border: w127 -> [w162]
              in-place-border: w126 -> [w161]
              in-place-border: w125 -> [w160]
              in-place-border: w124 -> [w159]
              in-place-border: w121 -> [w155]
              in-place-border: w120 -> [w154]
              in-place-border: w119 -> [w153]
              n74 = in-place-cluster #1(w123) -> ("Settings"=w156:T4)  [unwired: 1 out]
              n75 = Bundle By Name(cluster=w156, "Cycle Period"=500.0, "Ismatech"=w172, "Ismatech 3 Channel Settings"=w153, "Masterflex"=w171, "VICI Settings"=w170, "Output Device"=w167, "Manual Entry"=w169, "Tacmina Settings"=w168, "KNF SIMDOS Settings"=w166, "ASIA Pump C"=w165, "FLOM Settings"=w163, "Calibration Slope"=w162, "Calibration Y Intercept"=w159, "Pump Cal Enum"=w161, "SSI PR/LD Settings"=w160, "SSI P40 Settings"=w154, "Masterflex 75211 Settings"=w155) -> (w158:T4)
              n76 = in-place-cluster #1("Settings"=w158, "Process Name"="Module Name") -> (w122:T2)
            }
          }
          event Value Change {
            n77 = event-data() -> ()  [unwired: 1 in, 6 out]
            n78 = property on="ASIA Pump #" class="DigNum (strict)"() -> ("Value"=w185:i32)  [unwired: 2 in, 2 out]
            n79 = Greater Or Equal To 0?(x=w185) -> (x >= 0?=w187:bool)
            n80 = case shown="True" w187 {
              frame False {
                n81 = property on="OK Button" class="Bool"("DisabledEnum"=T22."Disabled and Grayed Out" ("Disabled")) -> ()  [unwired: 2 in, 2 out]
              }
              frame True {
                n82 = property on="OK Button" class="Bool"("DisabledEnum"=T22."Enabled" ("Disabled")) -> ()  [unwired: 2 in, 2 out]
              }
            }
          }
          event Value Change {
            n83 = event-data() -> ()  [unwired: 1 in, 1 out]
            n84 = property on="FLOM Settings" class="Clust (strict)"() -> ("Value"=w196:T13)  [unwired: 2 in, 2 out]
            n85 = Unbundle By Name(w196) -> ("VISA resource name"=w193:refnum<visa-resource-name>)
            n86 = local read "FLOM VISA Chosen"() -> (w194:bool)
            n87 = case shown="True" w194 {
              tunnel: w196 -> [w208 w216]
              tunnel: [w207 w216] -> w198
              tunnel: [w206 FALSE ("Initialized")] -> w197
              tunnel: w193 -> [w204 _]
              frame True {
                n88 = Empty String/Path?(string/path=w204) -> (empty?=w205:bool)
                n89 = case shown="False" w205 {
                  tunnel: w208 -> [w211 w213]
                  tunnel: [w210 w213] -> w207
                  tunnel: [w209 FALSE ("Initialized")] -> w206
                  frame False {
                    n90 = call "Initialize.vi"("FLOM Settings in"=w211) -> ("Initialized"=w209:bool, "FLOM Settings out"=w210:T13)  [unwired: 7 in, 2 out]
                  }
                  frame True {
                    n91 = One Button Dialog(message="Choose a non-zero Pump Number") -> ()  [unwired: 1 in, 1 out]
                  }
                }
              }
              frame False {
              }
            }
            n92 = case shown="False" w197 {
              frame False {
                n93 = control-ref of="OK Button"() -> (w218:refnum<vi>)
                n94 = One Button Dialog(message="No Pump Connected") -> ()  [unwired: 1 in, 1 out]
                n95 = property class="Bool"(reference=w218, "DisabledEnum"=T22."Disabled and Grayed Out" ("Disabled")) -> ()  [unwired: 1 in, 2 out]
              }
              frame True {
                n96 = control-ref of="OK Button"() -> (w220:refnum<vi>)
                n97 = property class="Bool"(reference=w220, "DisabledEnum"=T22."Enabled" ("Disabled")) -> ()  [unwired: 1 in, 2 out]
              }
            }
            n98 = Bundle By Name(cluster=w203, "Settings.FLOM Settings"=w198) -> (w202:T2)
            "FLOM Number Chosen" <- TRUE ("FLOM Number Chosen")
          }
          event Value Change {
            n99 = event-data() -> ("OldVal"=w230:refnum<visa-resource-name>)  [unwired: 1 in, 1 out]
            n100 = property on="FLOM Settings" class="Clust (strict)"() -> ("Value"=w227:T13)  [unwired: 2 in, 2 out]
            n101 = local read "FLOM Number Chosen"() -> (w225:bool)
            n102 = Unbundle By Name(w227) -> ("Pump Number"=w224:dbl)
            n103 = Not Equal To 0?(x=w224) -> (x != 0?=w223:bool)
            n104 = Or(x=w225, y=w223) -> (x .or. y?=w222:bool)
            n105 = VISA Close(VISA resource name=w230) -> (error out=w229:errorcluster)  [unwired: 1 in]
            n106 = case shown="True" w222 {
              tunnel: w227 -> [w242 w251]
              tunnel: [w241 w251] -> w231
              tunnel: w229 -> [w240 _]
              tunnel: [w239 FALSE ("Initialized")] -> w228
              tunnel: w224 -> [w238 _]
              frame True {
                n107 = Not Equal To 0?(x=w238) -> (x != 0?=w237:bool)
                n108 = case shown="True" w237 {
                  tunnel: w242 -> [w244 w249]
                  tunnel: [w244 w248] -> w241
                  tunnel: w240 -> [_ w247]
                  tunnel: [FALSE ("Initialized") w246] -> w239
                  frame False {
                    n109 = One Button Dialog(message="Choose a Pump Number") -> ()  [unwired: 1 in, 1 out]
                  }
                  frame True {
                    n110 = call "Initialize.vi"("error in (no error)"=w247, "FLOM Settings in"=w249) -> ("Initialized"=w246:bool, "FLOM Settings out"=w248:T13)  [unwired: 6 in, 2 out]
                  }
                }
              }
              frame False {
              }
            }
            n111 = case shown="False" w228 {
              frame False {
                n112 = control-ref of="OK Button"() -> (w253:refnum<vi>)
                n113 = One Button Dialog(message="No Pump Connected") -> ()  [unwired: 1 in, 1 out]
                n114 = property class="Bool"(reference=w253, "DisabledEnum"=T22."Disabled and Grayed Out" ("Disabled")) -> ()  [unwired: 1 in, 2 out]
              }
              frame True {
                n115 = control-ref of="OK Button"() -> (w255:refnum<vi>)
                n116 = property class="Bool"(reference=w255, "DisabledEnum"=T22."Enabled" ("Disabled")) -> ()  [unwired: 1 in, 2 out]
              }
            }
            n117 = Bundle By Name(cluster=w236, "Settings.FLOM Settings"=w231) -> (w235:T2)
            "FLOM VISA Chosen" <- TRUE ("FLOM VISA Chosen")
          }
          event Value Change {
            n118 = event-data() -> ("OldVal"=w264:refnum<visa-resource-name>)  [unwired: 1 in, 5 out]
            n119 = property on="Pump Configuration" class="Clust (strict)"() -> ("Value"=w265:T24)  [unwired: 2 in, 2 out]
            n120 = VISA Close(VISA resource name=w264, error in (no error)=w261) -> (error out=w266:errorcluster)
            n121 = Unbundle By Name(w265) -> ("Ismatech"=w268:T6)
            n122 = call "Initialize.vi"("error in (no error)"=w266, "Ismatech Settings"=w268) -> ("Initialized"=w257:bool, "Ismatech Settings"=w267:T6)  [unwired: 6 in, 2 out]
            n123 = case shown="False" w257 {
              tunnel: w267 -> [_ w277]
              tunnel: w263 -> [w272 w273]
              tunnel: [w272 w276] -> w262
              frame False {
                n124 = control-ref of="OK Button"() -> (w270:refnum<vi>)
                n125 = One Button Dialog(message="No Pump Connected") -> ()  [unwired: 1 in, 1 out]
                n126 = property class="Bool"(reference=w270, "DisabledEnum"=T22."Disabled and Grayed Out" ("Disabled")) -> ()  [unwired: 1 in, 2 out]
              }
              frame True {
                n127 = Bundle By Name(cluster=w273, "Settings.Ismatech"=w277) -> (w276:T2)
                n128 = control-ref of="OK Button"() -> (w274:refnum<vi>)
                n129 = property class="Bool"(reference=w274, "DisabledEnum"=T22."Enabled" ("Disabled")) -> ()  [unwired: 1 in, 2 out]
              }
            }
          }
          event Value Change {
            n130 = event-data() -> ("OldVal"=w281:T7, "NewVal"=w285:T7)  [unwired: 1 in, 4 out]
            n131 = Unbundle By Name(w281) -> ("VISA resource name"=w283:refnum<visa-resource-name>)
            n132 = Unbundle By Name(w285) -> ("VISA resource name"=w280:refnum<visa-resource-name>, "Pump Number"=w278:i16, "Channel Number"=w286:i16, "Simulated?"=w284:bool)
            n133 = Not Equal?(x=w283, y=w280) -> (x != y?=w282:bool)
            n134 = case shown="False" w282 {
              tunnel: w283 -> [_ w293]
              tunnel: [errorcluster {"status"=FALSE, "code"=0, "source"=""} ("error out") w292] -> w279
              frame False {
              }
              frame True {
                n135 = VISA Close(VISA resource name=w293) -> (error out=w292:errorcluster)  [unwired: 1 in]
              }
            }
            n136 = case shown="False" w284 {
              tunnel: w278 -> [w295 _]
              tunnel: w286 -> [w294 _]
              tunnel: w280 -> [w303 _]
              tunnel: w285 -> [w302 _]
              tunnel: w279 -> [w301 _]
              frame False {
                n137 = Empty String/Path?(string/path=w303) -> (empty?=w300:bool)
                n138 = Greater Than 0?(x=w294) -> (x > 0?=w297:bool)
                n139 = Not(x=w300) -> (.not. x?=w299:bool)
                n140 = Greater Than 0?(x=w295) -> (x > 0?=w298:bool)
                n141 = Compound Arithmetic op=AND(w299, w298, w297) -> (w296:bool)
                n142 = case shown="True" w296 {
                  tunnel: w302 -> [_ w311]
                  tunnel: w301 -> [_ w310]
                  tunnel: w295 -> [_ w307]
                  tunnel: w294 -> [_ w306]
                  frame False {
                    n143 = property on="OK Button" class="Bool"("DisabledEnum"=T22."Disabled and Grayed Out" ("Disabled")) -> ()  [unwired: 2 in, 2 out]
                  }
                  frame True {
                    n144 = call "Global Read.vi"("Pump Number"=w307) -> ("Initialized Channels"=w309:dbl[])  [unwired: 4 in, 6 out]
                    n145 = Search 1D Array(1D array=w309, element=w306) -> (index of element=w308:i32)  [unwired: 1 in]
                    n146 = Less Than 0?(x=w308) -> (x < 0?=w305:bool)
                    n147 = case shown="True" w305 {
                      tunnel: w311 -> [_ w318]
                      tunnel: w310 -> [_ w314]
                      frame False {
                        n148 = One Button Dialog(message="This channel has already been initialized elsewhere") -> ()  [unwired: 1 in, 1 out]
                        n149 = property on="OK Button" class="Bool"("DisabledEnum"=T22."Disabled and Grayed Out" ("Disabled")) -> ()  [unwired: 2 in, 2 out]
                      }
                      frame True {
                        n150 = call "Initialize.vi"("error in (no error)"=w314, "Ismatech 3 Channel Settings In"=w318) -> ("Initialized"=w315:bool, "Ismatech 3 Channel Settings Out"=w317:T7)  [unwired: 6 in, 2 out]
                        n151 = case shown="False" w315 {
                          tunnel: w317 -> [w320 w323]
                          tunnel: [w320 w323] -> w316
                          frame False {
                            n152 = One Button Dialog(message="No Pump Connected") -> ()  [unwired: 1 in, 1 out]
                            n153 = property on="OK Button" class="Bool"("DisabledEnum"=T22."Disabled and Grayed Out" ("Disabled")) -> ()  [unwired: 2 in, 2 out]
                          }
                          frame True {
                            n154 = property on="OK Button" class="Bool"("DisabledEnum"=T22."Enabled" ("Disabled")) -> ()  [unwired: 2 in, 2 out]
                          }
                        }
                        n155 = disable-structure shown="Disabled" {
                          disable-tunnel: w316 -> [w319 _]
                          frame Disabled {
                            n156 = call "Close.vi"("Ismatech 3 Channel Settings In"=w319) -> ()  [unwired: 8 in, 3 out]
                          }
                          frame Enabled {
                          }
                        }
                      }
                    }
                  }
                }
              }
              frame True {
                n157 = property on="OK Button" class="Bool"("DisabledEnum"=T22."Enabled" ("Disabled")) -> ()  [unwired: 2 in, 2 out]
              }
            }
          }
          event Value Change {
            n158 = event-data() -> ("OldVal"=w337:refnum<visa-resource-name>)  [unwired: 1 in, 5 out]
            n159 = property on="Pump Configuration" class="Clust (strict)"() -> ("Value"=w336:T24)  [unwired: 2 in, 2 out]
            n160 = VISA Close(VISA resource name=w337, error in (no error)=w333) -> (error out=w330:errorcluster)
            n161 = Unbundle By Name(w336) -> ("KNF SIMDOS Settings"=w332:T11)
            n162 = call "Initialize.vi"("error in (no error)"=w330, "KNF Settings In"=w332) -> ("Initialized"=w326:bool, "KNF Settings Out"=w331:T11)  [unwired: 6 in, 2 out]
            n163 = case shown="False" w326 {
              tunnel: w331 -> [_ w346]
              tunnel: w335 -> [w341 w345]
              tunnel: [w341 w344] -> w334
              frame False {
                n164 = control-ref of="OK Button"() -> (w339:refnum<vi>)
                n165 = One Button Dialog(message="No Pump Connected") -> ()  [unwired: 1 in, 1 out]
                n166 = property class="Bool"(reference=w339, "DisabledEnum"=T22."Disabled and Grayed Out" ("Disabled")) -> ()  [unwired: 1 in, 2 out]
              }
              frame True {
                n167 = Bundle By Name(cluster=w345, "Settings.KNF SIMDOS Settings"=w346) -> (w344:T2)
                n168 = control-ref of="OK Button"() -> (w342:refnum<vi>)
                n169 = property class="Bool"(reference=w342, "DisabledEnum"=T22."Enabled" ("Disabled")) -> ()  [unwired: 1 in, 2 out]
              }
            }
          }
          event Value Change {
            n170 = event-data() -> ("OldVal"=w358:refnum<visa-resource-name>)  [unwired: 1 in, 5 out]
            n171 = property on="Pump Configuration" class="Clust (strict)"() -> ("Value"=w355:T24)  [unwired: 2 in, 2 out]
            n172 = VISA Close(VISA resource name=w358, error in (no error)=w351) -> (error out=w354:errorcluster)
            n173 = Unbundle By Name(w355) -> ("Masterflex"=w357:T8)
            n174 = call "Initialize.vi"("error in (no error)"=w354, "Masterflex Settings in"=w357) -> ("Initialized"=w347:bool, "Masterflex Settings out"=w356:T8)  [unwired: 6 in, 2 out]
            n175 = case shown="False" w347 {
              tunnel: w356 -> [_ w367]
              tunnel: w353 -> [w362 w366]
              tunnel: [w362 w365] -> w352
              frame False {
                n176 = control-ref of="OK Button"() -> (w360:refnum<vi>)
                n177 = One Button Dialog(message="No Pump Connected") -> ()  [unwired: 1 in, 1 out]
                n178 = property class="Bool"(reference=w360, "DisabledEnum"=T22."Disabled and Grayed Out" ("Disabled")) -> ()  [unwired: 1 in, 2 out]
              }
              frame True {
                n179 = control-ref of="OK Button"() -> (w363:refnum<vi>)
                n180 = Bundle By Name(cluster=w366, "Settings.Masterflex"=w367) -> (w365:T2)
                n181 = property class="Bool"(reference=w363, "DisabledEnum"=T22."Enabled" ("Disabled")) -> ()  [unwired: 1 in, 2 out]
              }
            }
          }
          event Value Change {
            n182 = event-data() -> ("NewVal"=w373:T5)  [unwired: 1 in, 5 out]
            n183 = case "Selected Device" shown="\"Ismatec ISM 4308\"" w373 {
              tunnel: w372 -> [w384 w398 w412 w426 w440 w454 w468 w482 w503 w517 w531 w545]
              tunnel: [w384 w398 w412 w426 w440 w454 w468 w482 w503 w517 w531 w545] -> w371
              frame "Ismatec ISM 831C" {
                n184 = property on="VICI Settings" class="Clust (strict)"("Visible"=FALSE) -> ()  [unwired: 2 in, 2 out]
                n185 = property on="Tacmina Settings" class="Clust (strict)"("Visible"=FALSE) -> ()  [unwired: 2 in, 2 out]
                n186 = property on="Ismatech" class="Clust (strict)"("Visible"=TRUE) -> ()  [unwired: 2 in, 2 out]
                n187 = property on="Masterflex" class="Clust (strict)"("Visible"=FALSE) -> ()  [unwired: 2 in, 2 out]
                n188 = property on="FLOM Settings" class="Clust (strict)"("Visible"=FALSE) -> ()  [unwired: 2 in, 2 out]
                n189 = property on="KNF SIMDOS Settings" class="Clust (strict)"("Visible"=FALSE) -> ()  [unwired: 2 in, 2 out]
                n190 = property on="ASIA Pump C" class="Clust (strict)"("Visible"=FALSE) -> ()  [unwired: 2 in, 2 out]
                n191 = property on="Pump Calibration" class="Ring (strict)"("Visible"=FALSE) -> ()  [unwired: 2 in, 2 out]
                n192 = property on="SSI P40 Settings" class="Clust (strict)"("Visible"=FALSE) -> ()  [unwired: 2 in, 2 out]
                n193 = property on="Pump %" class="DigNum (strict)"("Caption.Text"="Pump %" ("Label.Text")) -> ()  [unwired: 2 in, 2 out]
                n194 = property on="SSI PR/LD Settings" class="Clust (strict)"("Visible"=FALSE) -> ()  [unwired: 2 in, 2 out]
                n195 = property on="Masterflex 75211 Settings" class="Clust (strict)"("Visible"=FALSE) -> ()  [unwired: 2 in, 2 out]
                n196 = property on="Ismatech 3 Channel Settings" class="Clust (strict)"("Visible"=FALSE) -> ()  [unwired: 2 in, 2 out]
              }
              frame "Ismatec ISM 4308" {
                n197 = property on="VICI Settings" class="Clust (strict)"("Visible"=FALSE) -> ()  [unwired: 2 in, 2 out]
                n198 = property on="Tacmina Settings" class="Clust (strict)"("Visible"=FALSE) -> ()  [unwired: 2 in, 2 out]
                n199 = property on="Ismatech" class="Clust (strict)"("Visible"=FALSE) -> ()  [unwired: 2 in, 2 out]
                n200 = property on="Masterflex" class="Clust (strict)"("Visible"=FALSE) -> ()  [unwired: 2 in, 2 out]
                n201 = property on="FLOM Settings" class="Clust (strict)"("Visible"=FALSE) -> ()  [unwired: 2 in, 2 out]
                n202 = property on="KNF SIMDOS Settings" class="Clust (strict)"("Visible"=FALSE) -> ()  [unwired: 2 in, 2 out]
                n203 = property on="ASIA Pump C" class="Clust (strict)"("Visible"=FALSE) -> ()  [unwired: 2 in, 2 out]
                n204 = property on="Pump Calibration" class="Ring (strict)"("Visible"=TRUE) -> ()  [unwired: 2 in, 2 out]
                n205 = property on="SSI P40 Settings" class="Clust (strict)"("Visible"=FALSE) -> ()  [unwired: 2 in, 2 out]
                n206 = property on="Pump %" class="DigNum (strict)"("Caption.Text"="ml/min" ("Label.Text")) -> ()  [unwired: 2 in, 2 out]
                n207 = property on="SSI PR/LD Settings" class="Clust (strict)"("Visible"=FALSE) -> ()  [unwired: 2 in, 2 out]
                n208 = property on="Masterflex 75211 Settings" class="Clust (strict)"("Visible"=FALSE) -> ()  [unwired: 2 in, 2 out]
                n209 = property on="Ismatech 3 Channel Settings" class="Clust (strict)"("Visible"=TRUE) -> ()  [unwired: 2 in, 2 out]
              }
              frame "Masterflex 7550-30" {
                n210 = property on="VICI Settings" class="Clust (strict)"("Visible"=FALSE) -> ()  [unwired: 2 in, 2 out]
                n211 = property on="Ismatech 3 Channel Settings" class="Clust (strict)"("Visible"=FALSE) -> ()  [unwired: 2 in, 2 out]
                n212 = property on="Ismatech" class="Clust (strict)"("Visible"=FALSE) -> ()  [unwired: 2 in, 2 out]
                n213 = property on="Masterflex" class="Clust (strict)"("Visible"=TRUE) -> ()  [unwired: 2 in, 2 out]
                n214 = property on="FLOM Settings" class="Clust (strict)"("Visible"=FALSE) -> ()  [unwired: 2 in, 2 out]
                n215 = property on="Pump Calibration" class="Ring (strict)"("Visible"=FALSE) -> ()  [unwired: 2 in, 2 out]
                n216 = property on="ASIA Pump C" class="Clust (strict)"("Visible"=FALSE) -> ()  [unwired: 2 in, 2 out]
                n217 = property on="KNF SIMDOS Settings" class="Clust (strict)"("Visible"=FALSE) -> ()  [unwired: 2 in, 2 out]
                n218 = property on="Tacmina Settings" class="Clust (strict)"("Visible"=FALSE) -> ()  [unwired: 2 in, 2 out]
                n219 = property on="Pump %" class="DigNum (strict)"("Caption.Text"="Pump %" ("Label.Text")) -> ()  [unwired: 2 in, 2 out]
                n220 = property on="SSI PR/LD Settings" class="Clust (strict)"("Visible"=FALSE) -> ()  [unwired: 2 in, 2 out]
                n221 = property on="Masterflex 75211 Settings" class="Clust (strict)"("Visible"=FALSE) -> ()  [unwired: 2 in, 2 out]
                n222 = property on="SSI P40 Settings" class="Clust (strict)"("Visible"=FALSE) -> ()  [unwired: 2 in, 2 out]
              }
              frame "VICI" {
                n223 = property on="KNF SIMDOS Settings" class="Clust (strict)"("Visible"=FALSE) -> ()  [unwired: 2 in, 2 out]
                n224 = property on="VICI Settings" class="Clust (strict)"("Visible"=TRUE) -> ()  [unwired: 2 in, 2 out]
                n225 = property on="Ismatech" class="Clust (strict)"("Visible"=FALSE) -> ()  [unwired: 2 in, 2 out]
                n226 = property on="Masterflex" class="Clust (strict)"("Visible"=FALSE) -> ()  [unwired: 2 in, 2 out]
                n227 = property on="ASIA Pump C" class="Clust (strict)"("Visible"=FALSE) -> ()  [unwired: 2 in, 2 out]
                n228 = property on="FLOM Settings" class="Clust (strict)"("Visible"=FALSE) -> ()  [unwired: 2 in, 2 out]
                n229 = property on="Pump Calibration" class="Ring (strict)"("Visible"=TRUE) -> ()  [unwired: 2 in, 2 out]
                n230 = property on="Ismatech 3 Channel Settings" class="Clust (strict)"("Visible"=FALSE) -> ()  [unwired: 2 in, 2 out]
                n231 = property on="Tacmina Settings" class="Clust (strict)"("Visible"=FALSE) -> ()  [unwired: 2 in, 2 out]
                n232 = property on="Pump %" class="DigNum (strict)"("Caption.Text"="ml/min" ("Label.Text")) -> ()  [unwired: 2 in, 2 out]
                n233 = property on="SSI PR/LD Settings" class="Clust (strict)"("Visible"=FALSE) -> ()  [unwired: 2 in, 2 out]
                n234 = property on="Masterflex 75211 Settings" class="Clust (strict)"("Visible"=FALSE) -> ()  [unwired: 2 in, 2 out]
                n235 = property on="SSI P40 Settings" class="Clust (strict)"("Visible"=FALSE) -> ()  [unwired: 2 in, 2 out]
              }
              frame "Tacmina QI" {
                n236 = property on="Tacmina Settings" class="Clust (strict)"("Visible"=TRUE) -> ()  [unwired: 2 in, 2 out]
                n237 = property on="VICI Settings" class="Clust (strict)"("Visible"=FALSE) -> ()  [unwired: 2 in, 2 out]
                n238 = property on="Ismatech" class="Clust (strict)"("Visible"=FALSE) -> ()  [unwired: 2 in, 2 out]
                n239 = property on="Masterflex" class="Clust (strict)"("Visible"=FALSE) -> ()  [unwired: 2 in, 2 out]
                n240 = property on="FLOM Settings" class="Clust (strict)"("Visible"=FALSE) -> ()  [unwired: 2 in, 2 out]
                n241 = property on="Pump Calibration" class="Ring (strict)"("Visible"=TRUE) -> ()  [unwired: 2 in, 2 out]
                n242 = property on="KNF SIMDOS Settings" class="Clust (strict)"("Visible"=FALSE) -> ()  [unwired: 2 in, 2 out]
                n243 = property on="ASIA Pump C" class="Clust (strict)"("Visible"=FALSE) -> ()  [unwired: 2 in, 2 out]
                n244 = property on="SSI P40 Settings" class="Clust (strict)"("Visible"=FALSE) -> ()  [unwired: 2 in, 2 out]
                n245 = property on="Pump %" class="DigNum (strict)"("Caption.Text"="ml/min" ("Label.Text")) -> ()  [unwired: 2 in, 2 out]
                n246 = property on="SSI PR/LD Settings" class="Clust (strict)"("Visible"=FALSE) -> ()  [unwired: 2 in, 2 out]
                n247 = property on="Masterflex 75211 Settings" class="Clust (strict)"("Visible"=FALSE) -> ()  [unwired: 2 in, 2 out]
                n248 = property on="Ismatech 3 Channel Settings" class="Clust (strict)"("Visible"=FALSE) -> ()  [unwired: 2 in, 2 out]
              }
              frame "Default", Default {
                n249 = property on="Tacmina Settings" class="Clust (strict)"("Visible"=FALSE) -> ()  [unwired: 2 in, 2 out]
                n250 = property on="VICI Settings" class="Clust (strict)"("Visible"=FALSE) -> ()  [unwired: 2 in, 2 out]
                n251 = property on="Ismatech" class="Clust (strict)"("Visible"=FALSE) -> ()  [unwired: 2 in, 2 out]
                n252 = property on="Masterflex" class="Clust (strict)"("Visible"=FALSE) -> ()  [unwired: 2 in, 2 out]
                n253 = property on="FLOM Settings" class="Clust (strict)"("Visible"=FALSE) -> ()  [unwired: 2 in, 2 out]
                n254 = property on="KNF SIMDOS Settings" class="Clust (strict)"("Visible"=FALSE) -> ()  [unwired: 2 in, 2 out]
                n255 = property on="ASIA Pump C" class="Clust (strict)"("Visible"=FALSE) -> ()  [unwired: 2 in, 2 out]
                n256 = property on="Pump Calibration" class="Ring (strict)"("Visible"=FALSE) -> ()  [unwired: 2 in, 2 out]
                n257 = property on="SSI P40 Settings" class="Clust (strict)"("Visible"=FALSE) -> ()  [unwired: 2 in, 2 out]
                n258 = property on="Pump %" class="DigNum (strict)"("Caption.Text"="Pump %" ("Label.Text")) -> ()  [unwired: 2 in, 2 out]
                n259 = property on="SSI PR/LD Settings" class="Clust (strict)"("Visible"=FALSE) -> ()  [unwired: 2 in, 2 out]
                n260 = property on="Masterflex 75211 Settings" class="Clust (strict)"("Visible"=FALSE) -> ()  [unwired: 2 in, 2 out]
                n261 = property on="Ismatech 3 Channel Settings" class="Clust (strict)"("Visible"=FALSE) -> ()  [unwired: 2 in, 2 out]
              }
              frame "KNF SIMDOS" {
                n262 = property on="VICI Settings" class="Clust (strict)"("Visible"=FALSE) -> ()  [unwired: 2 in, 2 out]
                n263 = property on="Ismatech" class="Clust (strict)"("Visible"=FALSE) -> ()  [unwired: 2 in, 2 out]
                n264 = property on="Masterflex" class="Clust (strict)"("Visible"=FALSE) -> ()  [unwired: 2 in, 2 out]
                n265 = property on="SSI P40 Settings" class="Clust (strict)"("Visible"=FALSE) -> ()  [unwired: 2 in, 2 out]
                n266 = property on="FLOM Settings" class="Clust (strict)"("Visible"=FALSE) -> ()  [unwired: 2 in, 2 out]
                n267 = property on="KNF SIMDOS Settings" class="Clust (strict)"("Visible"=TRUE) -> ()  [unwired: 2 in, 2 out]
                n268 = property on="ASIA Pump C" class="Clust (strict)"("Visible"=FALSE) -> ()  [unwired: 2 in, 2 out]
                n269 = property on="Pump Calibration" class="Ring (strict)"("Visible"=FALSE) -> ()  [unwired: 2 in, 2 out]
                n270 = property on="Tacmina Settings" class="Clust (strict)"("Visible"=FALSE) -> ()  [unwired: 2 in, 2 out]
                n271 = property on="Pump %" class="DigNum (strict)"("Caption.Text"="Pump %" ("Label.Text")) -> ()  [unwired: 2 in, 2 out]
                n272 = property on="SSI PR/LD Settings" class="Clust (strict)"("Visible"=FALSE) -> ()  [unwired: 2 in, 2 out]
                n273 = property on="Masterflex 75211 Settings" class="Clust (strict)"("Visible"=FALSE) -> ()  [unwired: 2 in, 2 out]
                n274 = property on="Ismatech 3 Channel Settings" class="Clust (strict)"("Visible"=FALSE) -> ()  [unwired: 2 in, 2 out]
              }
              frame "ASIA Type C" {
                n275 = Unbundle By Name(w482) -> ("Settings.ASIA Pump C.ASIA Pump #"=w481:i32)
                n276 = property on="SSI PR/LD Settings" class="Clust (strict)"("Visible"=FALSE) -> ()  [unwired: 2 in, 2 out]
                n277 = property on="KNF SIMDOS Settings" class="Clust (strict)"("Visible"=FALSE) -> ()  [unwired: 2 in, 2 out]
                n278 = property on="VICI Settings" class="Clust (strict)"("Visible"=FALSE) -> ()  [unwired: 2 in, 2 out]
                n279 = property on="Ismatech" class="Clust (strict)"("Visible"=FALSE) -> ()  [unwired: 2 in, 2 out]
                n280 = property on="Masterflex" class="Clust (strict)"("Visible"=FALSE) -> ()  [unwired: 2 in, 2 out]
                n281 = property on="ASIA Pump C" class="Clust (strict)"("Visible"=TRUE) -> ()  [unwired: 2 in, 2 out]
                n282 = property on="FLOM Settings" class="Clust (strict)"("Visible"=FALSE) -> ()  [unwired: 2 in, 2 out]
                n283 = property on="Pump Calibration" class="Ring (strict)"("Visible"=FALSE) -> ()  [unwired: 2 in, 2 out]
                n284 = property on="Masterflex 75211 Settings" class="Clust (strict)"("Visible"=FALSE) -> ()  [unwired: 2 in, 2 out]
                n285 = property on="SSI P40 Settings" class="Clust (strict)"("Visible"=FALSE) -> ()  [unwired: 2 in, 2 out]
                n286 = property on="Ismatech 3 Channel Settings" class="Clust (strict)"("Visible"=FALSE) -> ()  [unwired: 2 in, 2 out]
                n287 = Greater Or Equal To 0?(x=w481) -> (x >= 0?=w480:bool)
                n288 = case shown="False" w480 {
                  frame False {
                    n289 = property on="OK Button" class="Bool"("DisabledEnum"=T22."Disabled and Grayed Out" ("Disabled")) -> ()  [unwired: 2 in, 2 out]
                  }
                  frame True {
                    n290 = property on="OK Button" class="Bool"("DisabledEnum"=T22."Enabled" ("Disabled")) -> ()  [unwired: 2 in, 2 out]
                  }
                }
                n291 = property on="Pump %" class="DigNum (strict)"("Caption.Text"="ml/min" ("Label.Text")) -> ()  [unwired: 2 in, 2 out]
                n292 = property on="Tacmina Settings" class="Clust (strict)"("Visible"=FALSE) -> ()  [unwired: 2 in, 2 out]
              }
              frame "FLOM UI-22-11" {
                n293 = property on="VICI Settings" class="Clust (strict)"("Visible"=FALSE) -> ()  [unwired: 2 in, 2 out]
                n294 = property on="Ismatech" class="Clust (strict)"("Visible"=FALSE) -> ()  [unwired: 2 in, 2 out]
                n295 = property on="Masterflex" class="Clust (strict)"("Visible"=FALSE) -> ()  [unwired: 2 in, 2 out]
                n296 = property on="KNF SIMDOS Settings" class="Clust (strict)"("Visible"=FALSE) -> ()  [unwired: 2 in, 2 out]
                n297 = property on="Pump Calibration" class="Ring (strict)"("Visible"=FALSE) -> ()  [unwired: 2 in, 2 out]
                n298 = property on="ASIA Pump C" class="Clust (strict)"("Visible"=FALSE) -> ()  [unwired: 2 in, 2 out]
                n299 = property on="FLOM Settings" class="Clust (strict)"("Visible"=TRUE) -> ()  [unwired: 2 in, 2 out]
                n300 = property on="SSI PR/LD Settings" class="Clust (strict)"("Visible"=FALSE) -> ()  [unwired: 2 in, 2 out]
                n301 = property on="Ismatech 3 Channel Settings" class="Clust (strict)"("Visible"=FALSE) -> ()  [unwired: 2 in, 2 out]
                n302 = property on="Masterflex 75211 Settings" class="Clust (strict)"("Visible"=FALSE) -> ()  [unwired: 2 in, 2 out]
                n303 = property on="Tacmina Settings" class="Clust (strict)"("Visible"=FALSE) -> ()  [unwired: 2 in, 2 out]
                n304 = property on="SSI P40 Settings" class="Clust (strict)"("Visible"=FALSE) -> ()  [unwired: 2 in, 2 out]
                n305 = property on="Pump %" class="DigNum (strict)"("Caption.Text"="ml/min" ("Label.Text")) -> ()  [unwired: 2 in, 2 out]
              }
              frame "SSI PR/LD" {
                n306 = property on="VICI Settings" class="Clust (strict)"("Visible"=FALSE) -> ()  [unwired: 2 in, 2 out]
                n307 = property on="SSI P40 Settings" class="Clust (strict)"("Visible"=FALSE) -> ()  [unwired: 2 in, 2 out]
                n308 = property on="Ismatech" class="Clust (strict)"("Visible"=FALSE) -> ()  [unwired: 2 in, 2 out]
                n309 = property on="Masterflex" class="Clust (strict)"("Visible"=FALSE) -> ()  [unwired: 2 in, 2 out]
                n310 = property on="KNF SIMDOS Settings" class="Clust (strict)"("Visible"=FALSE) -> ()  [unwired: 2 in, 2 out]
                n311 = property on="FLOM Settings" class="Clust (strict)"("Visible"=FALSE) -> ()  [unwired: 2 in, 2 out]
                n312 = property on="Ismatech 3 Channel Settings" class="Clust (strict)"("Visible"=FALSE) -> ()  [unwired: 2 in, 2 out]
                n313 = property on="ASIA Pump C" class="Clust (strict)"("Visible"=FALSE) -> ()  [unwired: 2 in, 2 out]
                n314 = property on="Pump Calibration" class="Ring (strict)"("Visible"=FALSE) -> ()  [unwired: 2 in, 2 out]
                n315 = property on="Tacmina Settings" class="Clust (strict)"("Visible"=FALSE) -> ()  [unwired: 2 in, 2 out]
                n316 = property on="Pump %" class="DigNum (strict)"("Caption.Text"="ml/min" ("Label.Text")) -> ()  [unwired: 2 in, 2 out]
                n317 = property on="SSI PR/LD Settings" class="Clust (strict)"("Visible"=TRUE) -> ()  [unwired: 2 in, 2 out]
                n318 = property on="Masterflex 75211 Settings" class="Clust (strict)"("Visible"=FALSE) -> ()  [unwired: 2 in, 2 out]
              }
              frame "SSI P40" {
                n319 = property on="VICI Settings" class="Clust (strict)"("Visible"=FALSE) -> ()  [unwired: 2 in, 2 out]
                n320 = property on="Ismatech 3 Channel Settings" class="Clust (strict)"("Visible"=FALSE) -> ()  [unwired: 2 in, 2 out]
                n321 = property on="Ismatech" class="Clust (strict)"("Visible"=FALSE) -> ()  [unwired: 2 in, 2 out]
                n322 = property on="Masterflex" class="Clust (strict)"("Visible"=FALSE) -> ()  [unwired: 2 in, 2 out]
                n323 = property on="KNF SIMDOS Settings" class="Clust (strict)"("Visible"=FALSE) -> ()  [unwired: 2 in, 2 out]
                n324 = property on="FLOM Settings" class="Clust (strict)"("Visible"=FALSE) -> ()  [unwired: 2 in, 2 out]
                n325 = property on="ASIA Pump C" class="Clust (strict)"("Visible"=FALSE) -> ()  [unwired: 2 in, 2 out]
                n326 = property on="Pump Calibration" class="Ring (strict)"("Visible"=FALSE) -> ()  [unwired: 2 in, 2 out]
                n327 = property on="Tacmina Settings" class="Clust (strict)"("Visible"=FALSE) -> ()  [unwired: 2 in, 2 out]
                n328 = property on="SSI P40 Settings" class="Clust (strict)"("Visible"=TRUE) -> ()  [unwired: 2 in, 2 out]
                n329 = property on="Pump %" class="DigNum (strict)"("Caption.Text"="ml/min" ("Label.Text")) -> ()  [unwired: 2 in, 2 out]
                n330 = property on="SSI PR/LD Settings" class="Clust (strict)"("Visible"=FALSE) -> ()  [unwired: 2 in, 2 out]
                n331 = property on="Masterflex 75211 Settings" class="Clust (strict)"("Visible"=FALSE) -> ()  [unwired: 2 in, 2 out]
              }
              frame "Masterflex 75211-70" {
                n332 = property on="VICI Settings" class="Clust (strict)"("Visible"=FALSE) -> ()  [unwired: 2 in, 2 out]
                n333 = property on="SSI P40 Settings" class="Clust (strict)"("Visible"=FALSE) -> ()  [unwired: 2 in, 2 out]
                n334 = property on="Ismatech" class="Clust (strict)"("Visible"=FALSE) -> ()  [unwired: 2 in, 2 out]
                n335 = property on="Masterflex" class="Clust (strict)"("Visible"=FALSE) -> ()  [unwired: 2 in, 2 out]
                n336 = property on="FLOM Settings" class="Clust (strict)"("Visible"=FALSE) -> ()  [unwired: 2 in, 2 out]
                n337 = property on="ASIA Pump C" class="Clust (strict)"("Visible"=FALSE) -> ()  [unwired: 2 in, 2 out]
                n338 = property on="Pump Calibration" class="Ring (strict)"("Visible"=TRUE) -> ()  [unwired: 2 in, 2 out]
                n339 = property on="Ismatech 3 Channel Settings" class="Clust (strict)"("Visible"=FALSE) -> ()  [unwired: 2 in, 2 out]
                n340 = property on="Tacmina Settings" class="Clust (strict)"("Visible"=FALSE) -> ()  [unwired: 2 in, 2 out]
                n341 = property on="Pump %" class="DigNum (strict)"("Caption.Text"="ml/min" ("Label.Text")) -> ()  [unwired: 2 in, 2 out]
                n342 = property on="SSI PR/LD Settings" class="Clust (strict)"("Visible"=FALSE) -> ()  [unwired: 2 in, 2 out]
                n343 = property on="Masterflex 75211 Settings" class="Clust (strict)"("Visible"=TRUE) -> ()  [unwired: 2 in, 2 out]
                n344 = property on="KNF SIMDOS Settings" class="Clust (strict)"("Visible"=FALSE) -> ()  [unwired: 2 in, 2 out]
              }
            }
          }
          event Value Change {
            n345 = event-data() -> ()  [unwired: 1 in, 6 out]
            n346 = property on="Pump Configuration" class="Clust (strict)"() -> ("Value"=w554:T24)  [unwired: 2 in, 2 out]
            n347 = Unbundle By Name(w554) -> ("SSI PR/LD Settings"=w555:T14)
            n348 = call "Initialize.vi"("error in (no error)"=w551, "SSI PR Settings In"=w555) -> ("Initialized"=w546:bool, "SSI PR Settings Out"=w547:T14)  [unwired: 6 in, 2 out]
            n349 = case shown="False" w546 {
              tunnel: w547 -> [_ w564]
              tunnel: w553 -> [w559 w563]
              tunnel: [w559 w562] -> w552
              frame False {
                n350 = control-ref of="OK Button"() -> (w557:refnum<vi>)
                n351 = One Button Dialog(message="No Pump Connected") -> ()  [unwired: 1 in, 1 out]
                n352 = property class="Bool"(reference=w557, "DisabledEnum"=T22."Disabled and Grayed Out" ("Disabled")) -> ()  [unwired: 1 in, 2 out]
              }
              frame True {
                n353 = Bundle By Name(cluster=w563, "Settings.SSI PR/LD Settings"=w564) -> (w562:T2)
                n354 = control-ref of="OK Button"() -> (w560:refnum<vi>)
                n355 = property class="Bool"(reference=w560, "DisabledEnum"=T22."Enabled" ("Disabled")) -> ()  [unwired: 1 in, 2 out]
              }
            }
          }
          event Value Change {
            n356 = event-data() -> ()  [unwired: 1 in, 6 out]
            n357 = property on="Pump Configuration" class="Clust (strict)"() -> ("Value"=w574:T24)  [unwired: 2 in, 2 out]
            n358 = Unbundle By Name(w574) -> ("SSI P40 Settings"=w568:T19)
            n359 = call "Initialize P40.vi"("error in (no error)"=w567, "SSI P40 Settings In"=w568) -> ("Initialized"=w566:bool, "SSI P40 Settings Out"=w565:T19)  [unwired: 6 in, 2 out]
            n360 = case shown="False" w566 {
              tunnel: w565 -> [_ w583]
              tunnel: w573 -> [w578 w582]
              tunnel: [w578 w581] -> w572
              frame False {
                n361 = control-ref of="OK Button"() -> (w576:refnum<vi>)
                n362 = One Button Dialog(message="No Pump Connected") -> ()  [unwired: 1 in, 1 out]
                n363 = property class="Bool"(reference=w576, "DisabledEnum"=T22."Disabled and Grayed Out" ("Disabled")) -> ()  [unwired: 1 in, 2 out]
              }
              frame True {
                n364 = Bundle By Name(cluster=w582, "Settings.SSI PR/LD Settings"=w583) -> (w581:T2)
                n365 = control-ref of="OK Button"() -> (w579:refnum<vi>)
                n366 = property class="Bool"(reference=w579, "DisabledEnum"=T22."Enabled" ("Disabled")) -> ()  [unwired: 1 in, 2 out]
              }
            }
          }
          event Value Change {
            n367 = event-data() -> ()  [unwired: 1 in, 6 out]
            n368 = property on="Pump Configuration" class="Clust (strict)"() -> ("Value"=w591:T24)  [unwired: 2 in, 2 out]
            n369 = Unbundle By Name(w591) -> ("Tacmina Settings"=w588:T10)
            n370 = call "Initialize.vi"("Tacmina Settings in"=w588) -> ("Initialized"=w584:bool, "Tacmina Settings out"=w592:T10)  [unwired: 8 in, 1 out]
            n371 = case shown="True" w584 {
              frame False {
                n372 = control-ref of="OK Button"() -> (w594:refnum<vi>)
                n373 = One Button Dialog(message="No Pump Connected") -> ()  [unwired: 1 in, 1 out]
                n374 = property class="Bool"(reference=w594, "DisabledEnum"=T22."Disabled and Grayed Out" ("Disabled")) -> ()  [unwired: 1 in, 2 out]
              }
              frame True {
                n375 = control-ref of="OK Button"() -> (w596:refnum<vi>)
                n376 = property class="Bool"(reference=w596, "DisabledEnum"=T22."Enabled" ("Disabled")) -> ()  [unwired: 1 in, 2 out]
              }
            }
            n377 = Bundle By Name(cluster=w590, "Settings.Tacmina Settings"=w592) -> (w589:T2)
          }
          event Value Change {
            n378 = event-data() -> ()  [unwired: 1 in, 6 out]
            n379 = property on="Pump Configuration" class="Clust (strict)"() -> ("Value"=w606:T24)  [unwired: 2 in, 2 out]
            n380 = Unbundle By Name(w606) -> ("Masterflex 75211 Settings"=w600:T15)
            n381 = call "Initialize.vi"("Masterflex 75211 Settings"=w600) -> ("Initialized"=w598:bool, "Masterflex 75211 Settings"=w599:T15)  [unwired: 8 in, 1 out]
            n382 = case shown="True" w598 {
              frame False {
                n383 = control-ref of="OK Button"() -> (w608:refnum<vi>)
                n384 = One Button Dialog(message="No Pump Connected") -> ()  [unwired: 1 in, 1 out]
                n385 = property class="Bool"(reference=w608, "DisabledEnum"=T22."Disabled and Grayed Out" ("Disabled")) -> ()  [unwired: 1 in, 2 out]
              }
              frame True {
                n386 = control-ref of="OK Button"() -> (w610:refnum<vi>)
                n387 = property class="Bool"(reference=w610, "DisabledEnum"=T22."Enabled" ("Disabled")) -> ()  [unwired: 1 in, 2 out]
              }
            }
            n388 = Bundle By Name(cluster=w605, "Settings.Masterflex 75211 Settings"=w599) -> (w604:T2)
          }
          event Value Change {
            n389 = event-data() -> ()  [unwired: 1 in, 1 out]
            n390 = property on="Pump Configuration" class="Clust (strict)"() -> ("Value"=w618:T24)  [unwired: 2 in, 2 out]
            n391 = Unbundle By Name(w618) -> ("VICI Settings"=w619:T9)
            n392 = case shown="True" w614 {
              tunnel: w619 -> [_ w626]
              tunnel: w617 -> [w620 w624]
              tunnel: [w620 w623] -> w616
              tunnel: w615 -> [_ w622]
              frame False {
              }
              frame True {
                n393 = call "Initialize.vi"("error in (no error)"=w622, "VICI Settings"=w626) -> ("Initialized"=w621:bool, "VICI Settings"=w625:T9)  [unwired: 6 in, 2 out]
                n394 = case shown="False" w621 {
                  tunnel: w625 -> [_ w635]
                  tunnel: w624 -> [w630 w634]
                  tunnel: [w630 w633] -> w623
                  frame False {
                    n395 = control-ref of="OK Button"() -> (w628:refnum<vi>)
                    n396 = One Button Dialog(message="No Pump Connected") -> ()  [unwired: 1 in, 1 out]
                    n397 = property class="Bool"(reference=w628, "DisabledEnum"=T22."Disabled and Grayed Out" ("Disabled")) -> ()  [unwired: 1 in, 2 out]
                  }
                  frame True {
                    n398 = Bundle By Name(cluster=w634, "Settings.VICI Settings"=w635) -> (w633:T2)
                    n399 = control-ref of="OK Button"() -> (w631:refnum<vi>)
                    n400 = property class="Bool"(reference=w631, "DisabledEnum"=T22."Enabled" ("Disabled")) -> ()  [unwired: 1 in, 2 out]
                  }
                }
              }
            }
          }
          event Value Change {
            n401 = event-data() -> ("NewVal"=w636:bool)  [unwired: 1 in, 5 out]
            n402 = case shown="True" w636 {
              frame False {
              }
              frame True {
                n403 = control-ref of="OK Button"() -> (w642:refnum<vi>)
                n404 = property class="Bool"(reference=w642, "DisabledEnum"=T22."Enabled" ("Disabled")) -> ()  [unwired: 1 in, 2 out]
              }
            }
          }
          event Value Change {
            n405 = event-data() -> ("OldVal"=w649:refnum<visa-resource-name>)  [unwired: 1 in, 5 out]
            n406 = property on="Pump Configuration" class="Clust (strict)"() -> ("Value"=w650:T24)  [unwired: 2 in, 2 out]
            n407 = VISA Close(VISA resource name=w649, error in (no error)=w646) -> (error out=w651:errorcluster)
            n408 = Unbundle By Name(w650) -> ("VICI Settings"=w652:T9)
            n409 = case shown="True" w645 {
              tunnel: w652 -> [_ w659]
              tunnel: w651 -> [_ w657]
              tunnel: w648 -> [w653 w656]
              tunnel: [w653 w655] -> w647
              frame False {
              }
              frame True {
                n410 = call "Initialize.vi"("error in (no error)"=w657, "VICI Settings"=w659) -> ("Initialized"=w654:bool, "VICI Settings"=w658:T9)  [unwired: 6 in, 2 out]
                n411 = case shown="False" w654 {
                  tunnel: w658 -> [_ w668]
                  tunnel: w656 -> [w663 w667]
                  tunnel: [w663 w666] -> w655
                  frame False {
                    n412 = control-ref of="OK Button"() -> (w661:refnum<vi>)
                    n413 = property class="Bool"(reference=w661, "DisabledEnum"=T22."Disabled and Grayed Out" ("Disabled")) -> ()  [unwired: 1 in, 2 out]
                    n414 = One Button Dialog(message="No Pump Connected") -> ()  [unwired: 1 in, 1 out]
                  }
                  frame True {
                    n415 = Bundle By Name(cluster=w667, "Settings.VICI Settings"=w668) -> (w666:T2)
                    n416 = control-ref of="OK Button"() -> (w664:refnum<vi>)
                    n417 = property class="Bool"(reference=w664, "DisabledEnum"=T22."Enabled" ("Disabled")) -> ()  [unwired: 1 in, 2 out]
                  }
                }
              }
            }
          }
          event Value Change {
            n418 = event-data() -> ()  [unwired: 1 in, 6 out]
            n419 = control-ref of="Start"() -> (w674:refnum<vi>)
            n420 = control-ref of="Stop"() -> (w673:refnum<vi>)
            n421 = Build Array(w674) -> (w676:refnum<vi>[])
            n422 = Build Array(w673) -> (w678:refnum<vi>[])
            n423 = call "Set Enable State on Multiple Controls.vi"("Enable?"=FALSE, "Controls"=w676) -> ()  [unwired: 10 in]
            n424 = call "Set Enable State on Multiple Controls.vi"("Enable?"=TRUE, "Controls"=w678) -> ()  [unwired: 10 in]
          }
          event Value Change {
            n425 = event-data() -> ()  [unwired: 1 in, 6 out]
            n426 = control-ref of="Start"() -> (w684:refnum<vi>)
            n427 = control-ref of="Stop"() -> (w683:refnum<vi>)
            n428 = Build Array(w684) -> (w688:refnum<vi>[])
            n429 = Build Array(w683) -> (w686:refnum<vi>[])
            n430 = call "Set Enable State on Multiple Controls.vi"("Enable?"=TRUE, "Controls"=w688) -> ()  [unwired: 10 in]
            n431 = call "Set Enable State on Multiple Controls.vi"("Enable?"=FALSE, "Controls"=w686) -> ()  [unwired: 10 in]
          }
          event Value Change {
            n432 = event-data() -> ("NewVal"=w690:bool)  [unwired: 1 in, 5 out]
            n433 = Equal?(x=w690, y=TRUE) -> (x = y?=w689:bool)
            n434 = case shown="True" w689 {
              frame False {
              }
              frame True {
                n435 = property on="OK Button" class="Bool"("DisabledEnum"=T22."Enabled" ("Disabled")) -> ()  [unwired: 2 in, 2 out]
              }
            }
          }
        }
      }
      n436 = case shown="True" w24 {
        tunnel: w23 -> [w697 w698]
        tunnel: [_ w699] -> w32
        tunnel: [w697 w698] -> w33
        frame False {
        }
        frame True {
          # "Write settings back to XML"
          n437 = Flatten To XML(anything=w698) -> (xml string=w700:string)
          n438 = call "Get Config File Path.vi"() -> ("XML File Path"=w701:path)  [unwired: 10 in, 1 out]
          n439 = call-poly <vilib>:"Write to XML File.vi"("XML Input"=w700, "XML File Path"=w701) -> ("error out"=w699:errorcluster)  [unwired: 7 in, 2 out]
        }
      }
      n440 = case shown="\"Measuring\", Default" w28 {
        frame "Idle", "Paused" {
          n441 = control-ref of="Start"() -> (w36:refnum<vi>)
          n442 = control-ref of="Stop"() -> (w38:refnum<vi>)
          n443 = Build Array(w36) -> (w40:refnum<vi>[])
          n444 = Build Array(w38) -> (w37:refnum<vi>[])
          n445 = call "Set Enable State on Multiple Controls.vi"("Enable?"=TRUE, "Controls"=w40) -> ()  [unwired: 10 in]
          n446 = call "Set Enable State on Multiple Controls.vi"("Enable?"=FALSE, "Controls"=w37) -> ()  [unwired: 10 in]
        }
        frame "Measuring", Default {
          n447 = control-ref of="Stop"() -> (w42:refnum<vi>)
          n448 = control-ref of="Start"() -> (w43:refnum<vi>)
          n449 = Build Array(w42) -> (w46:refnum<vi>[])
          n450 = Build Array(w43) -> (w44:refnum<vi>[])
          n451 = call "Set Enable State on Multiple Controls.vi"("Enable?"=TRUE, "Controls"=w46) -> ()  [unwired: 10 in]
          n452 = call "Set Enable State on Multiple Controls.vi"("Enable?"=FALSE, "Controls"=w44) -> ()  [unwired: 10 in]
        }
      }
    }
    frame Error {
    }
  }
  "UI Refresh Needed?" <- w12
  "error out" <- w13
  "Cancelled?" <- w11
  "Pump Module Config Out" <- w7
